vi "20191023_KEK_HEX5_events.vi"() -> ()   [LabVIEW 2017]
uses:
  <vilib>/DAQmx/create/channels.llb/DAQmx Create Channel (AI-Voltage-Basic).vi
  <vilib>/DAQmx/create/channels.llb/DAQmx Create Channel (AO-Voltage-Basic).vi
  <vilib>/DAQmx/miscellaneous.llb/DAQmx Fill In Error Info.vi
  Lake Shore Cryotronics 218.lvlib
panel:
  in  "idx in":i32[](array[numeric])=[0, 1]
  out "Cycle #":i32=68
  out "current time":timestamp=timestamp(3644898422.6679497 s since 1904-01-01)
  in  "stop":bool
  in  "Tab Control":T1(tab)=enum."LSI CHs"
  out "ref LSI-D":refnum<file>
  in  "DAQ IN: P_4HeIN":tag="Dev1/ai16"
  in  "max_P4HeIN":dbl=5.0
  in  "min_P4HeIN":dbl
  in  "DAQ IN: BARA":tag="Dev1/ai7"
  in  "VISA LSI218 DOWN":refnum<visa-resource-name>="GPIB0::11::INSTR"
  in  "DAQ OUT ON?":bool
  out "ref DAQ":refnum<file>
  in  "max_OUT":dbl=5.0
  in  "min_OUT":dbl
  in  "max_FM3":dbl=5.0
  in  "min_FM3":dbl
  in  "max_FM4":dbl=5.0
  in  "min_FM4":dbl
  in  "max_dP3":dbl=5.0
  in  "min_dP3":dbl
  in  "max_dP4":dbl=5.0
  in  "min_dP4":dbl
  in  "max_LM":dbl=0.15
  in  "min_LM":dbl
  in  "max_P":dbl=5.0
  in  "min_P":dbl
  in  "DAQ IN: FM (3He)":tag="Dev1/ai6"
  in  "DAQ IN: FM (4He)":tag="Dev1/ai5"
  in  "DAQ IN: ƒ¢P (3He)":tag="Dev1/ai4"
  in  "DAQ IN: He-level":tag="Dev1/ai2"
  in  "DAQ IN: ƒ¢P (4He)":tag="Dev1/ai3"
  in  "DAQ IN: P (4He coil out)":tag="Dev1/ai1"
  in  "CSV filename suffix":string="TEST_"
  in  "base path":path=path "C:/Users/TUCAN_rcnp/Desktop/Labview/KEK_20191023_HEX5/TEST"
  out "ref LSI-U":refnum<file>
  in  "VISA LSI218 UP":refnum<visa-resource-name>="GPIB0::3::INSTR"
  in  "DAQ OUT":tag="Dev1/ao0"
  in  "sample #":i32=5
  out "error out \n(LSIU)":errorcluster
  out "error out\n(file creation)":errorcluster
  out "error out\n(DAQ config)":errorcluster
  out "error out\n(DAQ OUT)":errorcluster
  out "error out \n(DAQ IN)":errorcluster
  out "error out \n(record LSIU)":errorcluster
  out "error out \n(record DAQ)":errorcluster
  out "error out DAQ close":errorcluster
  out "error out \n(LSID)":errorcluster
  in  "max_BARA":dbl=5.0
  in  "min_BARA":dbl
  in  "min_P3HeOUT":dbl
  in  "max_P3HeOUT":dbl=5.0
  in  "DAQ IN: P_3HeOUT":tag="Dev1/ai17"
  out "error out \n(record LSID)":errorcluster
  out "errors plot cosmetic 1":errorcluster[](array[cluster])
  out "error plot content":errorcluster
  out "error plot cosmetic 2":errorcluster
  in  "LSI-D CH":string[](array[string])=["D1", "D2", "D3", "D4", "D5", "D6", "D7", "D8"]
  in  "NI DAQ AIN labels":string[](array[string])=["P_4KRES_COILIN", "LM", "DP_3He", "DP_4He", "FM_4He", "FM_3He", "P_4KRES_BARA", "P_4He_IN", "P_3He_OUT"]
  in  "LSI-U CH labels":string[](array[string])=["4K_res", "HEX_liq_IN", "HEX_liq_OUT", "1K_pot", "HEX_gas_IN", "HEX_gas_OUT", "JT_IN", "JT_OUT"]
  in  "LSI-D CH labels":string[](array[string])=["D1", "D2", "D3", "DISABLED", "D5", "D6", "D7", "D8"]
  in  "LSI-U CH":string[](array[string])=["U1", "U2", "U3", "U4", "U5", "U6", "U7", "U8"]
  in  "DAQ CH":string[](array[string])=["Q1", "Q2", "Q3", "Q4", "Q5", "Q6", "Q7", "Q8", "Q9"]
  out "D idx":i32[](array[numeric])=[0, 1]
  out "LSI-U CH indic,":string[](array[string])=["U1", "U2", "U3", "U4", "U5", "U6", "U7", "U8"]
  out "LSI-U out":dbl[](array[numeric])=[305.92, 296.12, 291.08, 301.5, 302.08, 302.37, 301.36, 300.38]
  in  "GraphU1 SEL":i32[](array[numeric])=[0, 1]
  out "LSI-D out":dbl[](array[numeric])=[305.92, 296.12, 291.08, 301.5, 302.08, 302.37, 301.36, 300.38]
  out "LSI-D CH indic.":string[](array[string])=["U1", "U2", "U3", "U4", "U5", "U6", "U7", "U8"]
  in  "GraphU2 SEL":i32[](array[numeric])=[2, 3, 4]
  in  "GraphU3 SEL":i32[](array[numeric])=[5, 6, 6]
  in  "GraphD1 SEL":i32[](array[numeric])=[0, 1]
  in  "GraphD2 SEL":i32[](array[numeric])=[2, 3, 4]
  in  "GraphD3 SEL":i32[](array[numeric])=[5, 6, 6]
  out "LSI-D Grpah 1":cluster{dbl[], dbl[]}[](graph)=[{[3644898082.6645026, 3644898087.663789, 3644898092.6640744, 3644898097.66436, 3644898102.6646466, 3644898107.663933, 3644898112.6642184, 3644898117.664504, 3644898122.66379, 3644898127.664076, 3644898132.6643624, 3644898137.665648, 3644898142.6649346, 3644898147.66522, 3644898152.6655064, 3644898157.664792, 3644898162.665078, 3644898167.665364, 3644898172.6656504, 3644898177.664936, 3644898182.665222, 3644898187.665508, 3644898192.6647944, 3644898197.66508, 3644898202.6663666, 3644898207.666652, 3644898212.6659384, 3644898217.666224, 3644898222.6665106, 3644898227.665796, 3644898232.6660824, 3644898237.667368, 3644898242.6676545, 3644898247.66694, 3644898252.6672263, 3644898257.667512, 3644898262.6667986, 3644898267.667084, 3644898272.6673694, 3644898277.667656, 3644898282.6669426, 3644898287.667228, 3644898292.6675134, 3644898297.6678, 3644898302.6680865, 3644898307.668372, 3644898312.668658, 3644898317.667944, 3644898322.6682296, 3644898327.668516, 3644898332.6678014, 3644898337.668088, 3644898342.6683736, 3644898347.66866, 3644898352.6679454, 3644898357.668232, 3644898362.6685176, 3644898367.667804, 3644898372.6680894, 3644898377.668376, 3644898382.6686616, 3644898387.667948, 3644898392.6682334, 3644898397.66852, 3644898402.6678057, 3644898407.6680913, 3644898412.6683774, 3644898417.668664, 3644898422.6679497], [305.66, 305.96, 305.22, 305.33, 305.78, 305.05, 305.43, 306.1, 305.47, 305.83, 305.61, 305.97, 305.69, 305.75, 305.82, 305.82, 305.69, 305.52, 305.52, 306.2, 306.15, 305.92, 305.78, 305.61, 305.73, 305.41, 305.57, 306.24, 306.43, 305.83, 305.97, 306.01, 306.34, 305.78, 305.78, 306.48, 306.2, 306.2, 305.47, 305.96, 305.57, 305.97, 305.83, 305.83, 306.06, 305.92, 305.66, 305.82, 305.64, 305.57, 305.78, 305.73, 306.17, 305.83, 305.9, 306.15, 305.43, 305.87, 306.24, 306.04, 305.82, 306.06, 305.52, 305.75, 306.04, 306.06, 305.48, 305.75, 305.92]}, {[3644898082.6645026, 3644898087.663789, 3644898092.6640744, 3644898097.66436, 3644898102.6646466, 3644898107.663933, 3644898112.6642184, 3644898117.664504, 3644898122.66379, 3644898127.664076, 3644898132.6643624, 3644898137.665648, 3644898142.6649346, 3644898147.66522, 3644898152.6655064, 3644898157.664792, 3644898162.665078, 3644898167.665364, 3644898172.6656504, 3644898177.664936, 3644898182.665222, 3644898187.665508, 3644898192.6647944, 3644898197.66508, 3644898202.6663666, 3644898207.666652, 3644898212.6659384, 3644898217.666224, 3644898222.6665106, 3644898227.665796, 3644898232.6660824, 3644898237.667368, 3644898242.6676545, 3644898247.66694, 3644898252.6672263, 3644898257.667512, 3644898262.6667986, 3644898267.667084, 3644898272.6673694, 3644898277.667656, 3644898282.6669426, 3644898287.667228, 3644898292.6675134, 3644898297.6678, 3644898302.6680865, 3644898307.668372, 3644898312.668658, 3644898317.667944, 3644898322.6682296, 3644898327.668516, 3644898332.6678014, 3644898337.668088, 3644898342.6683736, 3644898347.66866, 3644898352.6679454, 3644898357.668232, 3644898362.6685176, 3644898367.667804, 3644898372.6680894, 3644898377.668376, 3644898382.6686616, 3644898387.667948, 3644898392.6682334, 3644898397.66852, 3644898402.6678057, 3644898407.6680913, 3644898412.6683774, 3644898417.668664, 3644898422.6679497], [296.0, 296.1, 295.89, 295.78, 295.94, 295.91, 295.97, 296.12, 296.01, 296.1, 296.01, 296.2, 296.14, 296.06, 296.16, 296.08, 295.89, 295.97, 296.06, 296.03, 296.09, 295.99, 295.89, 295.85, 295.93, 295.74, 295.91, 296.21, 296.04, 296.14, 296.12, 295.91, 296.2, 295.91, 295.87, 296.09, 296.19, 295.91, 296.03, 296.12, 295.94, 296.03, 295.97, 296.01, 296.08, 295.89, 295.91, 295.97, 296.03, 295.81, 295.91, 296.1, 296.15, 296.05, 296.15, 296.24, 295.82, 295.81, 296.14, 296.24, 295.97, 296.06, 295.74, 295.95, 296.08, 295.94, 295.91, 295.91, 296.12]}, {[3644898082.6645026, 3644898087.663789, 3644898092.6640744, 3644898097.66436, 3644898102.6646466, 3644898107.663933, 3644898112.6642184, 3644898117.664504, 3644898122.66379, 3644898127.664076, 3644898132.6643624, 3644898137.665648, 3644898142.6649346, 3644898147.66522, 3644898152.6655064, 3644898157.664792, 3644898162.665078, 3644898167.665364, 3644898172.6656504, 3644898177.664936, 3644898182.665222, 3644898187.665508, 3644898192.6647944, 3644898197.66508, 3644898202.6663666, 3644898207.666652, 3644898212.6659384, 3644898217.666224, 3644898222.6665106, 3644898227.665796, 3644898232.6660824, 3644898237.667368, 3644898242.6676545, 3644898247.66694, 3644898252.6672263, 3644898257.667512, 3644898262.6667986, 3644898267.667084, 3644898272.6673694, 3644898277.667656, 3644898282.6669426, 3644898287.667228, 3644898292.6675134, 3644898297.6678, 3644898302.6680865, 3644898307.668372, 3644898312.668658, 3644898317.667944, 3644898322.6682296, 3644898327.668516, 3644898332.6678014, 3644898337.668088, 3644898342.6683736, 3644898347.66866, 3644898352.6679454, 3644898357.668232, 3644898362.6685176, 3644898367.667804, 3644898372.6680894, 3644898377.668376, 3644898382.6686616, 3644898387.667948, 3644898392.6682334, 3644898397.66852, 3644898402.6678057, 3644898407.6680913, 3644898412.6683774, 3644898417.668664, 3644898422.6679497], [290.48, 291.09, 290.9, 291.1, 290.9, 290.9, 291.04, 291.04, 290.99, 290.93, 290.9, 291.31, 290.97, 291.13, 291.04, 291.12, 290.93, 290.69, 291.06, 291.27, 291.06, 291.04, 290.96, 291.09, 290.86, 290.95, 291.01, 291.18, 291.25, 291.18, 290.95, 291.08, 291.12, 290.97, 290.93, 291.09, 291.27, 291.02, 290.93, 291.08, 291.22, 291.12, 290.92, 290.69, 291.02, 291.02, 290.9, 290.86, 291.08, 290.88, 290.77, 291.01, 291.05, 291.1, 291.14, 290.99, 291.06, 290.9, 291.05, 291.31, 291.05, 291.06, 290.95, 290.99, 290.99, 290.9, 290.9, 290.96, 291.08]}]
  out "LSI-U Grpah 1":cluster{dbl[], dbl[]}[](graph)=[{[3644898082.6645026, 3644898087.663789, 3644898092.6640744, 3644898097.66436, 3644898102.6646466, 3644898107.663933, 3644898112.6642184, 3644898117.664504, 3644898122.66379, 3644898127.664076, 3644898132.6643624, 3644898137.665648, 3644898142.6649346, 3644898147.66522, 3644898152.6655064, 3644898157.664792, 3644898162.665078, 3644898167.665364, 3644898172.6656504, 3644898177.664936, 3644898182.665222, 3644898187.665508, 3644898192.6647944, 3644898197.66508, 3644898202.6663666, 3644898207.666652, 3644898212.6659384, 3644898217.666224, 3644898222.6665106, 3644898227.665796, 3644898232.6660824, 3644898237.667368, 3644898242.6676545, 3644898247.66694, 3644898252.6672263, 3644898257.667512, 3644898262.6667986, 3644898267.667084, 3644898272.6673694, 3644898277.667656, 3644898282.6669426, 3644898287.667228, 3644898292.6675134, 3644898297.6678, 3644898302.6680865, 3644898307.668372, 3644898312.668658, 3644898317.667944, 3644898322.6682296, 3644898327.668516, 3644898332.6678014, 3644898337.668088, 3644898342.6683736, 3644898347.66866, 3644898352.6679454, 3644898357.668232, 3644898362.6685176, 3644898367.667804, 3644898372.6680894, 3644898377.668376, 3644898382.6686616, 3644898387.667948, 3644898392.6682334, 3644898397.66852, 3644898402.6678057, 3644898407.6680913, 3644898412.6683774, 3644898417.668664, 3644898422.6679497], [305.66, 305.96, 305.22, 305.33, 305.78, 305.05, 305.43, 306.1, 305.47, 305.83, 305.61, 305.97, 305.69, 305.75, 305.82, 305.82, 305.69, 305.52, 305.52, 306.2, 306.15, 305.92, 305.78, 305.61, 305.73, 305.41, 305.57, 306.24, 306.43, 305.83, 305.97, 306.01, 306.34, 305.78, 305.78, 306.48, 306.2, 306.2, 305.47, 305.96, 305.57, 305.97, 305.83, 305.83, 306.06, 305.92, 305.66, 305.82, 305.64, 305.57, 305.78, 305.73, 306.17, 305.83, 305.9, 306.15, 305.43, 305.87, 306.24, 306.04, 305.82, 306.06, 305.52, 305.75, 306.04, 306.06, 305.48, 305.75, 305.92]}, {[3644898082.6645026, 3644898087.663789, 3644898092.6640744, 3644898097.66436, 3644898102.6646466, 3644898107.663933, 3644898112.6642184, 3644898117.664504, 3644898122.66379, 3644898127.664076, 3644898132.6643624, 3644898137.665648, 3644898142.6649346, 3644898147.66522, 3644898152.6655064, 3644898157.664792, 3644898162.665078, 3644898167.665364, 3644898172.6656504, 3644898177.664936, 3644898182.665222, 3644898187.665508, 3644898192.6647944, 3644898197.66508, 3644898202.6663666, 3644898207.666652, 3644898212.6659384, 3644898217.666224, 3644898222.6665106, 3644898227.665796, 3644898232.6660824, 3644898237.667368, 3644898242.6676545, 3644898247.66694, 3644898252.6672263, 3644898257.667512, 3644898262.6667986, 3644898267.667084, 3644898272.6673694, 3644898277.667656, 3644898282.6669426, 3644898287.667228, 3644898292.6675134, 3644898297.6678, 3644898302.6680865, 3644898307.668372, 3644898312.668658, 3644898317.667944, 3644898322.6682296, 3644898327.668516, 3644898332.6678014, 3644898337.668088, 3644898342.6683736, 3644898347.66866, 3644898352.6679454, 3644898357.668232, 3644898362.6685176, 3644898367.667804, 3644898372.6680894, 3644898377.668376, 3644898382.6686616, 3644898387.667948, 3644898392.6682334, 3644898397.66852, 3644898402.6678057, 3644898407.6680913, 3644898412.6683774, 3644898417.668664, 3644898422.6679497], [296.0, 296.1, 295.89, 295.78, 295.94, 295.91, 295.97, 296.12, 296.01, 296.1, 296.01, 296.2, 296.14, 296.06, 296.16, 296.08, 295.89, 295.97, 296.06, 296.03, 296.09, 295.99, 295.89, 295.85, 295.93, 295.74, 295.91, 296.21, 296.04, 296.14, 296.12, 295.91, 296.2, 295.91, 295.87, 296.09, 296.19, 295.91, 296.03, 296.12, 295.94, 296.03, 295.97, 296.01, 296.08, 295.89, 295.91, 295.97, 296.03, 295.81, 295.91, 296.1, 296.15, 296.05, 296.15, 296.24, 295.82, 295.81, 296.14, 296.24, 295.97, 296.06, 295.74, 295.95, 296.08, 295.94, 295.91, 295.91, 296.12]}, {[3644898082.6645026, 3644898087.663789, 3644898092.6640744, 3644898097.66436, 3644898102.6646466, 3644898107.663933, 3644898112.6642184, 3644898117.664504, 3644898122.66379, 3644898127.664076, 3644898132.6643624, 3644898137.665648, 3644898142.6649346, 3644898147.66522, 3644898152.6655064, 3644898157.664792, 3644898162.665078, 3644898167.665364, 3644898172.6656504, 3644898177.664936, 3644898182.665222, 3644898187.665508, 3644898192.6647944, 3644898197.66508, 3644898202.6663666, 3644898207.666652, 3644898212.6659384, 3644898217.666224, 3644898222.6665106, 3644898227.665796, 3644898232.6660824, 3644898237.667368, 3644898242.6676545, 3644898247.66694, 3644898252.6672263, 3644898257.667512, 3644898262.6667986, 3644898267.667084, 3644898272.6673694, 3644898277.667656, 3644898282.6669426, 3644898287.667228, 3644898292.6675134, 3644898297.6678, 3644898302.6680865, 3644898307.668372, 3644898312.668658, 3644898317.667944, 3644898322.6682296, 3644898327.668516, 3644898332.6678014, 3644898337.668088, 3644898342.6683736, 3644898347.66866, 3644898352.6679454, 3644898357.668232, 3644898362.6685176, 3644898367.667804, 3644898372.6680894, 3644898377.668376, 3644898382.6686616, 3644898387.667948, 3644898392.6682334, 3644898397.66852, 3644898402.6678057, 3644898407.6680913, 3644898412.6683774, 3644898417.668664, 3644898422.6679497], [290.48, 291.09, 290.9, 291.1, 290.9, 290.9, 291.04, 291.04, 290.99, 290.93, 290.9, 291.31, 290.97, 291.13, 291.04, 291.12, 290.93, 290.69, 291.06, 291.27, 291.06, 291.04, 290.96, 291.09, 290.86, 290.95, 291.01, 291.18, 291.25, 291.18, 290.95, 291.08, 291.12, 290.97, 290.93, 291.09, 291.27, 291.02, 290.93, 291.08, 291.22, 291.12, 290.92, 290.69, 291.02, 291.02, 290.9, 290.86, 291.08, 290.88, 290.77, 291.01, 291.05, 291.1, 291.14, 290.99, 291.06, 290.9, 291.05, 291.31, 291.05, 291.06, 290.95, 290.99, 290.99, 290.9, 290.9, 290.96, 291.08]}]
  out "LSI-D Grpah 2":cluster{dbl[], dbl[]}[](graph)=[{[3644898082.6645026, 3644898087.663789, 3644898092.6640744, 3644898097.66436, 3644898102.6646466, 3644898107.663933, 3644898112.6642184, 3644898117.664504, 3644898122.66379, 3644898127.664076, 3644898132.6643624, 3644898137.665648, 3644898142.6649346, 3644898147.66522, 3644898152.6655064, 3644898157.664792, 3644898162.665078, 3644898167.665364, 3644898172.6656504, 3644898177.664936, 3644898182.665222, 3644898187.665508, 3644898192.6647944, 3644898197.66508, 3644898202.6663666, 3644898207.666652, 3644898212.6659384, 3644898217.666224, 3644898222.6665106, 3644898227.665796, 3644898232.6660824, 3644898237.667368, 3644898242.6676545, 3644898247.66694, 3644898252.6672263, 3644898257.667512, 3644898262.6667986, 3644898267.667084, 3644898272.6673694, 3644898277.667656, 3644898282.6669426, 3644898287.667228, 3644898292.6675134, 3644898297.6678, 3644898302.6680865, 3644898307.668372, 3644898312.668658, 3644898317.667944, 3644898322.6682296, 3644898327.668516, 3644898332.6678014, 3644898337.668088, 3644898342.6683736, 3644898347.66866, 3644898352.6679454, 3644898357.668232, 3644898362.6685176, 3644898367.667804, 3644898372.6680894, 3644898377.668376, 3644898382.6686616, 3644898387.667948, 3644898392.6682334, 3644898397.66852, 3644898402.6678057, 3644898407.6680913, 3644898412.6683774, 3644898417.668664, 3644898422.6679497], [305.66, 305.96, 305.22, 305.33, 305.78, 305.05, 305.43, 306.1, 305.47, 305.83, 305.61, 305.97, 305.69, 305.75, 305.82, 305.82, 305.69, 305.52, 305.52, 306.2, 306.15, 305.92, 305.78, 305.61, 305.73, 305.41, 305.57, 306.24, 306.43, 305.83, 305.97, 306.01, 306.34, 305.78, 305.78, 306.48, 306.2, 306.2, 305.47, 305.96, 305.57, 305.97, 305.83, 305.83, 306.06, 305.92, 305.66, 305.82, 305.64, 305.57, 305.78, 305.73, 306.17, 305.83, 305.9, 306.15, 305.43, 305.87, 306.24, 306.04, 305.82, 306.06, 305.52, 305.75, 306.04, 306.06, 305.48, 305.75, 305.92]}, {[3644898082.6645026, 3644898087.663789, 3644898092.6640744, 3644898097.66436, 3644898102.6646466, 3644898107.663933, 3644898112.6642184, 3644898117.664504, 3644898122.66379, 3644898127.664076, 3644898132.6643624, 3644898137.665648, 3644898142.6649346, 3644898147.66522, 3644898152.6655064, 3644898157.664792, 3644898162.665078, 3644898167.665364, 3644898172.6656504, 3644898177.664936, 3644898182.665222, 3644898187.665508, 3644898192.6647944, 3644898197.66508, 3644898202.6663666, 3644898207.666652, 3644898212.6659384, 3644898217.666224, 3644898222.6665106, 3644898227.665796, 3644898232.6660824, 3644898237.667368, 3644898242.6676545, 3644898247.66694, 3644898252.6672263, 3644898257.667512, 3644898262.6667986, 3644898267.667084, 3644898272.6673694, 3644898277.667656, 3644898282.6669426, 3644898287.667228, 3644898292.6675134, 3644898297.6678, 3644898302.6680865, 3644898307.668372, 3644898312.668658, 3644898317.667944, 3644898322.6682296, 3644898327.668516, 3644898332.6678014, 3644898337.668088, 3644898342.6683736, 3644898347.66866, 3644898352.6679454, 3644898357.668232, 3644898362.6685176, 3644898367.667804, 3644898372.6680894, 3644898377.668376, 3644898382.6686616, 3644898387.667948, 3644898392.6682334, 3644898397.66852, 3644898402.6678057, 3644898407.6680913, 3644898412.6683774, 3644898417.668664, 3644898422.6679497], [296.0, 296.1, 295.89, 295.78, 295.94, 295.91, 295.97, 296.12, 296.01, 296.1, 296.01, 296.2, 296.14, 296.06, 296.16, 296.08, 295.89, 295.97, 296.06, 296.03, 296.09, 295.99, 295.89, 295.85, 295.93, 295.74, 295.91, 296.21, 296.04, 296.14, 296.12, 295.91, 296.2, 295.91, 295.87, 296.09, 296.19, 295.91, 296.03, 296.12, 295.94, 296.03, 295.97, 296.01, 296.08, 295.89, 295.91, 295.97, 296.03, 295.81, 295.91, 296.1, 296.15, 296.05, 296.15, 296.24, 295.82, 295.81, 296.14, 296.24, 295.97, 296.06, 295.74, 295.95, 296.08, 295.94, 295.91, 295.91, 296.12]}, {[3644898082.6645026, 3644898087.663789, 3644898092.6640744, 3644898097.66436, 3644898102.6646466, 3644898107.663933, 3644898112.6642184, 3644898117.664504, 3644898122.66379, 3644898127.664076, 3644898132.6643624, 3644898137.665648, 3644898142.6649346, 3644898147.66522, 3644898152.6655064, 3644898157.664792, 3644898162.665078, 3644898167.665364, 3644898172.6656504, 3644898177.664936, 3644898182.665222, 3644898187.665508, 3644898192.6647944, 3644898197.66508, 3644898202.6663666, 3644898207.666652, 3644898212.6659384, 3644898217.666224, 3644898222.6665106, 3644898227.665796, 3644898232.6660824, 3644898237.667368, 3644898242.6676545, 3644898247.66694, 3644898252.6672263, 3644898257.667512, 3644898262.6667986, 3644898267.667084, 3644898272.6673694, 3644898277.667656, 3644898282.6669426, 3644898287.667228, 3644898292.6675134, 3644898297.6678, 3644898302.6680865, 3644898307.668372, 3644898312.668658, 3644898317.667944, 3644898322.6682296, 3644898327.668516, 3644898332.6678014, 3644898337.668088, 3644898342.6683736, 3644898347.66866, 3644898352.6679454, 3644898357.668232, 3644898362.6685176, 3644898367.667804, 3644898372.6680894, 3644898377.668376, 3644898382.6686616, 3644898387.667948, 3644898392.6682334, 3644898397.66852, 3644898402.6678057, 3644898407.6680913, 3644898412.6683774, 3644898417.668664, 3644898422.6679497], [290.48, 291.09, 290.9, 291.1, 290.9, 290.9, 291.04, 291.04, 290.99, 290.93, 290.9, 291.31, 290.97, 291.13, 291.04, 291.12, 290.93, 290.69, 291.06, 291.27, 291.06, 291.04, 290.96, 291.09, 290.86, 290.95, 291.01, 291.18, 291.25, 291.18, 290.95, 291.08, 291.12, 290.97, 290.93, 291.09, 291.27, 291.02, 290.93, 291.08, 291.22, 291.12, 290.92, 290.69, 291.02, 291.02, 290.9, 290.86, 291.08, 290.88, 290.77, 291.01, 291.05, 291.1, 291.14, 290.99, 291.06, 290.9, 291.05, 291.31, 291.05, 291.06, 290.95, 290.99, 290.99, 290.9, 290.9, 290.96, 291.08]}]
  out "LSI-U Grpah 3":cluster{dbl[], dbl[]}[](graph)=[{[3644898082.6645026, 3644898087.663789, 3644898092.6640744, 3644898097.66436, 3644898102.6646466, 3644898107.663933, 3644898112.6642184, 3644898117.664504, 3644898122.66379, 3644898127.664076, 3644898132.6643624, 3644898137.665648, 3644898142.6649346, 3644898147.66522, 3644898152.6655064, 3644898157.664792, 3644898162.665078, 3644898167.665364, 3644898172.6656504, 3644898177.664936, 3644898182.665222, 3644898187.665508, 3644898192.6647944, 3644898197.66508, 3644898202.6663666, 3644898207.666652, 3644898212.6659384, 3644898217.666224, 3644898222.6665106, 3644898227.665796, 3644898232.6660824, 3644898237.667368, 3644898242.6676545, 3644898247.66694, 3644898252.6672263, 3644898257.667512, 3644898262.6667986, 3644898267.667084, 3644898272.6673694, 3644898277.667656, 3644898282.6669426, 3644898287.667228, 3644898292.6675134, 3644898297.6678, 3644898302.6680865, 3644898307.668372, 3644898312.668658, 3644898317.667944, 3644898322.6682296, 3644898327.668516, 3644898332.6678014, 3644898337.668088, 3644898342.6683736, 3644898347.66866, 3644898352.6679454, 3644898357.668232, 3644898362.6685176, 3644898367.667804, 3644898372.6680894, 3644898377.668376, 3644898382.6686616, 3644898387.667948, 3644898392.6682334, 3644898397.66852, 3644898402.6678057, 3644898407.6680913, 3644898412.6683774, 3644898417.668664, 3644898422.6679497], [305.66, 305.96, 305.22, 305.33, 305.78, 305.05, 305.43, 306.1, 305.47, 305.83, 305.61, 305.97, 305.69, 305.75, 305.82, 305.82, 305.69, 305.52, 305.52, 306.2, 306.15, 305.92, 305.78, 305.61, 305.73, 305.41, 305.57, 306.24, 306.43, 305.83, 305.97, 306.01, 306.34, 305.78, 305.78, 306.48, 306.2, 306.2, 305.47, 305.96, 305.57, 305.97, 305.83, 305.83, 306.06, 305.92, 305.66, 305.82, 305.64, 305.57, 305.78, 305.73, 306.17, 305.83, 305.9, 306.15, 305.43, 305.87, 306.24, 306.04, 305.82, 306.06, 305.52, 305.75, 306.04, 306.06, 305.48, 305.75, 305.92]}, {[3644898082.6645026, 3644898087.663789, 3644898092.6640744, 3644898097.66436, 3644898102.6646466, 3644898107.663933, 3644898112.6642184, 3644898117.664504, 3644898122.66379, 3644898127.664076, 3644898132.6643624, 3644898137.665648, 3644898142.6649346, 3644898147.66522, 3644898152.6655064, 3644898157.664792, 3644898162.665078, 3644898167.665364, 3644898172.6656504, 3644898177.664936, 3644898182.665222, 3644898187.665508, 3644898192.6647944, 3644898197.66508, 3644898202.6663666, 3644898207.666652, 3644898212.6659384, 3644898217.666224, 3644898222.6665106, 3644898227.665796, 3644898232.6660824, 3644898237.667368, 3644898242.6676545, 3644898247.66694, 3644898252.6672263, 3644898257.667512, 3644898262.6667986, 3644898267.667084, 3644898272.6673694, 3644898277.667656, 3644898282.6669426, 3644898287.667228, 3644898292.6675134, 3644898297.6678, 3644898302.6680865, 3644898307.668372, 3644898312.668658, 3644898317.667944, 3644898322.6682296, 3644898327.668516, 3644898332.6678014, 3644898337.668088, 3644898342.6683736, 3644898347.66866, 3644898352.6679454, 3644898357.668232, 3644898362.6685176, 3644898367.667804, 3644898372.6680894, 3644898377.668376, 3644898382.6686616, 3644898387.667948, 3644898392.6682334, 3644898397.66852, 3644898402.6678057, 3644898407.6680913, 3644898412.6683774, 3644898417.668664, 3644898422.6679497], [296.0, 296.1, 295.89, 295.78, 295.94, 295.91, 295.97, 296.12, 296.01, 296.1, 296.01, 296.2, 296.14, 296.06, 296.16, 296.08, 295.89, 295.97, 296.06, 296.03, 296.09, 295.99, 295.89, 295.85, 295.93, 295.74, 295.91, 296.21, 296.04, 296.14, 296.12, 295.91, 296.2, 295.91, 295.87, 296.09, 296.19, 295.91, 296.03, 296.12, 295.94, 296.03, 295.97, 296.01, 296.08, 295.89, 295.91, 295.97, 296.03, 295.81, 295.91, 296.1, 296.15, 296.05, 296.15, 296.24, 295.82, 295.81, 296.14, 296.24, 295.97, 296.06, 295.74, 295.95, 296.08, 295.94, 295.91, 295.91, 296.12]}, {[3644898082.6645026, 3644898087.663789, 3644898092.6640744, 3644898097.66436, 3644898102.6646466, 3644898107.663933, 3644898112.6642184, 3644898117.664504, 3644898122.66379, 3644898127.664076, 3644898132.6643624, 3644898137.665648, 3644898142.6649346, 3644898147.66522, 3644898152.6655064, 3644898157.664792, 3644898162.665078, 3644898167.665364, 3644898172.6656504, 3644898177.664936, 3644898182.665222, 3644898187.665508, 3644898192.6647944, 3644898197.66508, 3644898202.6663666, 3644898207.666652, 3644898212.6659384, 3644898217.666224, 3644898222.6665106, 3644898227.665796, 3644898232.6660824, 3644898237.667368, 3644898242.6676545, 3644898247.66694, 3644898252.6672263, 3644898257.667512, 3644898262.6667986, 3644898267.667084, 3644898272.6673694, 3644898277.667656, 3644898282.6669426, 3644898287.667228, 3644898292.6675134, 3644898297.6678, 3644898302.6680865, 3644898307.668372, 3644898312.668658, 3644898317.667944, 3644898322.6682296, 3644898327.668516, 3644898332.6678014, 3644898337.668088, 3644898342.6683736, 3644898347.66866, 3644898352.6679454, 3644898357.668232, 3644898362.6685176, 3644898367.667804, 3644898372.6680894, 3644898377.668376, 3644898382.6686616, 3644898387.667948, 3644898392.6682334, 3644898397.66852, 3644898402.6678057, 3644898407.6680913, 3644898412.6683774, 3644898417.668664, 3644898422.6679497], [290.48, 291.09, 290.9, 291.1, 290.9, 290.9, 291.04, 291.04, 290.99, 290.93, 290.9, 291.31, 290.97, 291.13, 291.04, 291.12, 290.93, 290.69, 291.06, 291.27, 291.06, 291.04, 290.96, 291.09, 290.86, 290.95, 291.01, 291.18, 291.25, 291.18, 290.95, 291.08, 291.12, 290.97, 290.93, 291.09, 291.27, 291.02, 290.93, 291.08, 291.22, 291.12, 290.92, 290.69, 291.02, 291.02, 290.9, 290.86, 291.08, 290.88, 290.77, 291.01, 291.05, 291.1, 291.14, 290.99, 291.06, 290.9, 291.05, 291.31, 291.05, 291.06, 290.95, 290.99, 290.99, 290.9, 290.9, 290.96, 291.08]}]
  out "LSI-U Grpah 2":cluster{dbl[], dbl[]}[](graph)=[{[3644898082.6645026, 3644898087.663789, 3644898092.6640744, 3644898097.66436, 3644898102.6646466, 3644898107.663933, 3644898112.6642184, 3644898117.664504, 3644898122.66379, 3644898127.664076, 3644898132.6643624, 3644898137.665648, 3644898142.6649346, 3644898147.66522, 3644898152.6655064, 3644898157.664792, 3644898162.665078, 3644898167.665364, 3644898172.6656504, 3644898177.664936, 3644898182.665222, 3644898187.665508, 3644898192.6647944, 3644898197.66508, 3644898202.6663666, 3644898207.666652, 3644898212.6659384, 3644898217.666224, 3644898222.6665106, 3644898227.665796, 3644898232.6660824, 3644898237.667368, 3644898242.6676545, 3644898247.66694, 3644898252.6672263, 3644898257.667512, 3644898262.6667986, 3644898267.667084, 3644898272.6673694, 3644898277.667656, 3644898282.6669426, 3644898287.667228, 3644898292.6675134, 3644898297.6678, 3644898302.6680865, 3644898307.668372, 3644898312.668658, 3644898317.667944, 3644898322.6682296, 3644898327.668516, 3644898332.6678014, 3644898337.668088, 3644898342.6683736, 3644898347.66866, 3644898352.6679454, 3644898357.668232, 3644898362.6685176, 3644898367.667804, 3644898372.6680894, 3644898377.668376, 3644898382.6686616, 3644898387.667948, 3644898392.6682334, 3644898397.66852, 3644898402.6678057, 3644898407.6680913, 3644898412.6683774, 3644898417.668664, 3644898422.6679497], [305.66, 305.96, 305.22, 305.33, 305.78, 305.05, 305.43, 306.1, 305.47, 305.83, 305.61, 305.97, 305.69, 305.75, 305.82, 305.82, 305.69, 305.52, 305.52, 306.2, 306.15, 305.92, 305.78, 305.61, 305.73, 305.41, 305.57, 306.24, 306.43, 305.83, 305.97, 306.01, 306.34, 305.78, 305.78, 306.48, 306.2, 306.2, 305.47, 305.96, 305.57, 305.97, 305.83, 305.83, 306.06, 305.92, 305.66, 305.82, 305.64, 305.57, 305.78, 305.73, 306.17, 305.83, 305.9, 306.15, 305.43, 305.87, 306.24, 306.04, 305.82, 306.06, 305.52, 305.75, 306.04, 306.06, 305.48, 305.75, 305.92]}, {[3644898082.6645026, 3644898087.663789, 3644898092.6640744, 3644898097.66436, 3644898102.6646466, 3644898107.663933, 3644898112.6642184, 3644898117.664504, 3644898122.66379, 3644898127.664076, 3644898132.6643624, 3644898137.665648, 3644898142.6649346, 3644898147.66522, 3644898152.6655064, 3644898157.664792, 3644898162.665078, 3644898167.665364, 3644898172.6656504, 3644898177.664936, 3644898182.665222, 3644898187.665508, 3644898192.6647944, 3644898197.66508, 3644898202.6663666, 3644898207.666652, 3644898212.6659384, 3644898217.666224, 3644898222.6665106, 3644898227.665796, 3644898232.6660824, 3644898237.667368, 3644898242.6676545, 3644898247.66694, 3644898252.6672263, 3644898257.667512, 3644898262.6667986, 3644898267.667084, 3644898272.6673694, 3644898277.667656, 3644898282.6669426, 3644898287.667228, 3644898292.6675134, 3644898297.6678, 3644898302.6680865, 3644898307.668372, 3644898312.668658, 3644898317.667944, 3644898322.6682296, 3644898327.668516, 3644898332.6678014, 3644898337.668088, 3644898342.6683736, 3644898347.66866, 3644898352.6679454, 3644898357.668232, 3644898362.6685176, 3644898367.667804, 3644898372.6680894, 3644898377.668376, 3644898382.6686616, 3644898387.667948, 3644898392.6682334, 3644898397.66852, 3644898402.6678057, 3644898407.6680913, 3644898412.6683774, 3644898417.668664, 3644898422.6679497], [296.0, 296.1, 295.89, 295.78, 295.94, 295.91, 295.97, 296.12, 296.01, 296.1, 296.01, 296.2, 296.14, 296.06, 296.16, 296.08, 295.89, 295.97, 296.06, 296.03, 296.09, 295.99, 295.89, 295.85, 295.93, 295.74, 295.91, 296.21, 296.04, 296.14, 296.12, 295.91, 296.2, 295.91, 295.87, 296.09, 296.19, 295.91, 296.03, 296.12, 295.94, 296.03, 295.97, 296.01, 296.08, 295.89, 295.91, 295.97, 296.03, 295.81, 295.91, 296.1, 296.15, 296.05, 296.15, 296.24, 295.82, 295.81, 296.14, 296.24, 295.97, 296.06, 295.74, 295.95, 296.08, 295.94, 295.91, 295.91, 296.12]}, {[3644898082.6645026, 3644898087.663789, 3644898092.6640744, 3644898097.66436, 3644898102.6646466, 3644898107.663933, 3644898112.6642184, 3644898117.664504, 3644898122.66379, 3644898127.664076, 3644898132.6643624, 3644898137.665648, 3644898142.6649346, 3644898147.66522, 3644898152.6655064, 3644898157.664792, 3644898162.665078, 3644898167.665364, 3644898172.6656504, 3644898177.664936, 3644898182.665222, 3644898187.665508, 3644898192.6647944, 3644898197.66508, 3644898202.6663666, 3644898207.666652, 3644898212.6659384, 3644898217.666224, 3644898222.6665106, 3644898227.665796, 3644898232.6660824, 3644898237.667368, 3644898242.6676545, 3644898247.66694, 3644898252.6672263, 3644898257.667512, 3644898262.6667986, 3644898267.667084, 3644898272.6673694, 3644898277.667656, 3644898282.6669426, 3644898287.667228, 3644898292.6675134, 3644898297.6678, 3644898302.6680865, 3644898307.668372, 3644898312.668658, 3644898317.667944, 3644898322.6682296, 3644898327.668516, 3644898332.6678014, 3644898337.668088, 3644898342.6683736, 3644898347.66866, 3644898352.6679454, 3644898357.668232, 3644898362.6685176, 3644898367.667804, 3644898372.6680894, 3644898377.668376, 3644898382.6686616, 3644898387.667948, 3644898392.6682334, 3644898397.66852, 3644898402.6678057, 3644898407.6680913, 3644898412.6683774, 3644898417.668664, 3644898422.6679497], [290.48, 291.09, 290.9, 291.1, 290.9, 290.9, 291.04, 291.04, 290.99, 290.93, 290.9, 291.31, 290.97, 291.13, 291.04, 291.12, 290.93, 290.69, 291.06, 291.27, 291.06, 291.04, 290.96, 291.09, 290.86, 290.95, 291.01, 291.18, 291.25, 291.18, 290.95, 291.08, 291.12, 290.97, 290.93, 291.09, 291.27, 291.02, 290.93, 291.08, 291.22, 291.12, 290.92, 290.69, 291.02, 291.02, 290.9, 290.86, 291.08, 290.88, 290.77, 291.01, 291.05, 291.1, 291.14, 290.99, 291.06, 290.9, 291.05, 291.31, 291.05, 291.06, 290.95, 290.99, 290.99, 290.9, 290.9, 290.96, 291.08]}]
  out "LSI-D Grpah 3":cluster{dbl[], dbl[]}[](graph)=[{[3644898082.6645026, 3644898087.663789, 3644898092.6640744, 3644898097.66436, 3644898102.6646466, 3644898107.663933, 3644898112.6642184, 3644898117.664504, 3644898122.66379, 3644898127.664076, 3644898132.6643624, 3644898137.665648, 3644898142.6649346, 3644898147.66522, 3644898152.6655064, 3644898157.664792, 3644898162.665078, 3644898167.665364, 3644898172.6656504, 3644898177.664936, 3644898182.665222, 3644898187.665508, 3644898192.6647944, 3644898197.66508, 3644898202.6663666, 3644898207.666652, 3644898212.6659384, 3644898217.666224, 3644898222.6665106, 3644898227.665796, 3644898232.6660824, 3644898237.667368, 3644898242.6676545, 3644898247.66694, 3644898252.6672263, 3644898257.667512, 3644898262.6667986, 3644898267.667084, 3644898272.6673694, 3644898277.667656, 3644898282.6669426, 3644898287.667228, 3644898292.6675134, 3644898297.6678, 3644898302.6680865, 3644898307.668372, 3644898312.668658, 3644898317.667944, 3644898322.6682296, 3644898327.668516, 3644898332.6678014, 3644898337.668088, 3644898342.6683736, 3644898347.66866, 3644898352.6679454, 3644898357.668232, 3644898362.6685176, 3644898367.667804, 3644898372.6680894, 3644898377.668376, 3644898382.6686616, 3644898387.667948, 3644898392.6682334, 3644898397.66852, 3644898402.6678057, 3644898407.6680913, 3644898412.6683774, 3644898417.668664, 3644898422.6679497], [305.66, 305.96, 305.22, 305.33, 305.78, 305.05, 305.43, 306.1, 305.47, 305.83, 305.61, 305.97, 305.69, 305.75, 305.82, 305.82, 305.69, 305.52, 305.52, 306.2, 306.15, 305.92, 305.78, 305.61, 305.73, 305.41, 305.57, 306.24, 306.43, 305.83, 305.97, 306.01, 306.34, 305.78, 305.78, 306.48, 306.2, 306.2, 305.47, 305.96, 305.57, 305.97, 305.83, 305.83, 306.06, 305.92, 305.66, 305.82, 305.64, 305.57, 305.78, 305.73, 306.17, 305.83, 305.9, 306.15, 305.43, 305.87, 306.24, 306.04, 305.82, 306.06, 305.52, 305.75, 306.04, 306.06, 305.48, 305.75, 305.92]}, {[3644898082.6645026, 3644898087.663789, 3644898092.6640744, 3644898097.66436, 3644898102.6646466, 3644898107.663933, 3644898112.6642184, 3644898117.664504, 3644898122.66379, 3644898127.664076, 3644898132.6643624, 3644898137.665648, 3644898142.6649346, 3644898147.66522, 3644898152.6655064, 3644898157.664792, 3644898162.665078, 3644898167.665364, 3644898172.6656504, 3644898177.664936, 3644898182.665222, 3644898187.665508, 3644898192.6647944, 3644898197.66508, 3644898202.6663666, 3644898207.666652, 3644898212.6659384, 3644898217.666224, 3644898222.6665106, 3644898227.665796, 3644898232.6660824, 3644898237.667368, 3644898242.6676545, 3644898247.66694, 3644898252.6672263, 3644898257.667512, 3644898262.6667986, 3644898267.667084, 3644898272.6673694, 3644898277.667656, 3644898282.6669426, 3644898287.667228, 3644898292.6675134, 3644898297.6678, 3644898302.6680865, 3644898307.668372, 3644898312.668658, 3644898317.667944, 3644898322.6682296, 3644898327.668516, 3644898332.6678014, 3644898337.668088, 3644898342.6683736, 3644898347.66866, 3644898352.6679454, 3644898357.668232, 3644898362.6685176, 3644898367.667804, 3644898372.6680894, 3644898377.668376, 3644898382.6686616, 3644898387.667948, 3644898392.6682334, 3644898397.66852, 3644898402.6678057, 3644898407.6680913, 3644898412.6683774, 3644898417.668664, 3644898422.6679497], [296.0, 296.1, 295.89, 295.78, 295.94, 295.91, 295.97, 296.12, 296.01, 296.1, 296.01, 296.2, 296.14, 296.06, 296.16, 296.08, 295.89, 295.97, 296.06, 296.03, 296.09, 295.99, 295.89, 295.85, 295.93, 295.74, 295.91, 296.21, 296.04, 296.14, 296.12, 295.91, 296.2, 295.91, 295.87, 296.09, 296.19, 295.91, 296.03, 296.12, 295.94, 296.03, 295.97, 296.01, 296.08, 295.89, 295.91, 295.97, 296.03, 295.81, 295.91, 296.1, 296.15, 296.05, 296.15, 296.24, 295.82, 295.81, 296.14, 296.24, 295.97, 296.06, 295.74, 295.95, 296.08, 295.94, 295.91, 295.91, 296.12]}, {[3644898082.6645026, 3644898087.663789, 3644898092.6640744, 3644898097.66436, 3644898102.6646466, 3644898107.663933, 3644898112.6642184, 3644898117.664504, 3644898122.66379, 3644898127.664076, 3644898132.6643624, 3644898137.665648, 3644898142.6649346, 3644898147.66522, 3644898152.6655064, 3644898157.664792, 3644898162.665078, 3644898167.665364, 3644898172.6656504, 3644898177.664936, 3644898182.665222, 3644898187.665508, 3644898192.6647944, 3644898197.66508, 3644898202.6663666, 3644898207.666652, 3644898212.6659384, 3644898217.666224, 3644898222.6665106, 3644898227.665796, 3644898232.6660824, 3644898237.667368, 3644898242.6676545, 3644898247.66694, 3644898252.6672263, 3644898257.667512, 3644898262.6667986, 3644898267.667084, 3644898272.6673694, 3644898277.667656, 3644898282.6669426, 3644898287.667228, 3644898292.6675134, 3644898297.6678, 3644898302.6680865, 3644898307.668372, 3644898312.668658, 3644898317.667944, 3644898322.6682296, 3644898327.668516, 3644898332.6678014, 3644898337.668088, 3644898342.6683736, 3644898347.66866, 3644898352.6679454, 3644898357.668232, 3644898362.6685176, 3644898367.667804, 3644898372.6680894, 3644898377.668376, 3644898382.6686616, 3644898387.667948, 3644898392.6682334, 3644898397.66852, 3644898402.6678057, 3644898407.6680913, 3644898412.6683774, 3644898417.668664, 3644898422.6679497], [290.48, 291.09, 290.9, 291.1, 290.9, 290.9, 291.04, 291.04, 290.99, 290.93, 290.9, 291.31, 290.97, 291.13, 291.04, 291.12, 290.93, 290.69, 291.06, 291.27, 291.06, 291.04, 290.96, 291.09, 290.86, 290.95, 291.01, 291.18, 291.25, 291.18, 290.95, 291.08, 291.12, 290.97, 290.93, 291.09, 291.27, 291.02, 290.93, 291.08, 291.22, 291.12, 290.92, 290.69, 291.02, 291.02, 290.9, 290.86, 291.08, 290.88, 290.77, 291.01, 291.05, 291.1, 291.14, 290.99, 291.06, 290.9, 291.05, 291.31, 291.05, 291.06, 290.95, 290.99, 290.99, 290.9, 290.9, 290.96, 291.08]}]
  out "U idx":i32[](array[numeric])=[0, 1]
  out "NI DAQ OUT":dbl[](array[numeric])=[-50013.24569663551, 15.025355709698363, -250.03334959533717, -250.04156931728906, -26.29672579614668, -0.7155199244462975, 103537.91205606361, -50000.0, -50000.0] format="%#_3f"
  out "NI-DAQ CH indic.":string[](array[string])=["U1", "U2", "U3", "U4", "U5", "U6", "U7", "U8"]
  out "Graph S. 1":cluster{dbl[], dbl[]}[](graph)
  in  "log/linear 4":bool
  in  "log/linear 1":bool
  out "Graph S. 3":cluster{dbl[], dbl[]}[](graph)
  in  "log/linear 6":bool
  in  "log/linear 3":bool
  in  "log/linear 2":bool
  out "Graph S. 6":cluster{dbl[], dbl[]}[](graph)
  out "Graph S. 5":cluster{dbl[], dbl[]}[](graph)
  in  "log/linear 5":bool
  in  "S.5 SEL":i32[](array[numeric])=[0, 2, 3]
  out "Graph S. 4":cluster{dbl[], dbl[]}[](graph)
  in  "S.1 SEL":i32[](array[numeric])=[0, 2]
  in  "S.2 SEL":i32[](array[numeric])=[1]
  out "Graph S. 2":cluster{dbl[], dbl[]}[](graph)
  in  "S.3 SEL":i32[](array[numeric])=[0, 2, 3]
  in  "S.4 SEL":i32[](array[numeric])=[0, 2, 3]
  in  "S.6 SEL":i32[](array[numeric])=[0, 2, 3]
  in  "DAQ OUT SET Volt":dbl[](array[numeric])=[2.0] format="%0.2f"
  out "DAQ OUT \nsample #":u32=1
  out "Q idx":i32[](array[numeric])=[0, 1]
  out "date/time string":string="20190702_164122_"
  in  "Wait (s)":i32=5
  # "Some time needed until program stops!"
  # "Record Config"
  # "VISA address"
  # "Error states"
  # "CH4 of LSI-D broken!"
  # "NI-DAQ config"
  # "Defines # of measurements \n taken for averaging"
  # "Inputs on this page have to be filled before the start of the program"
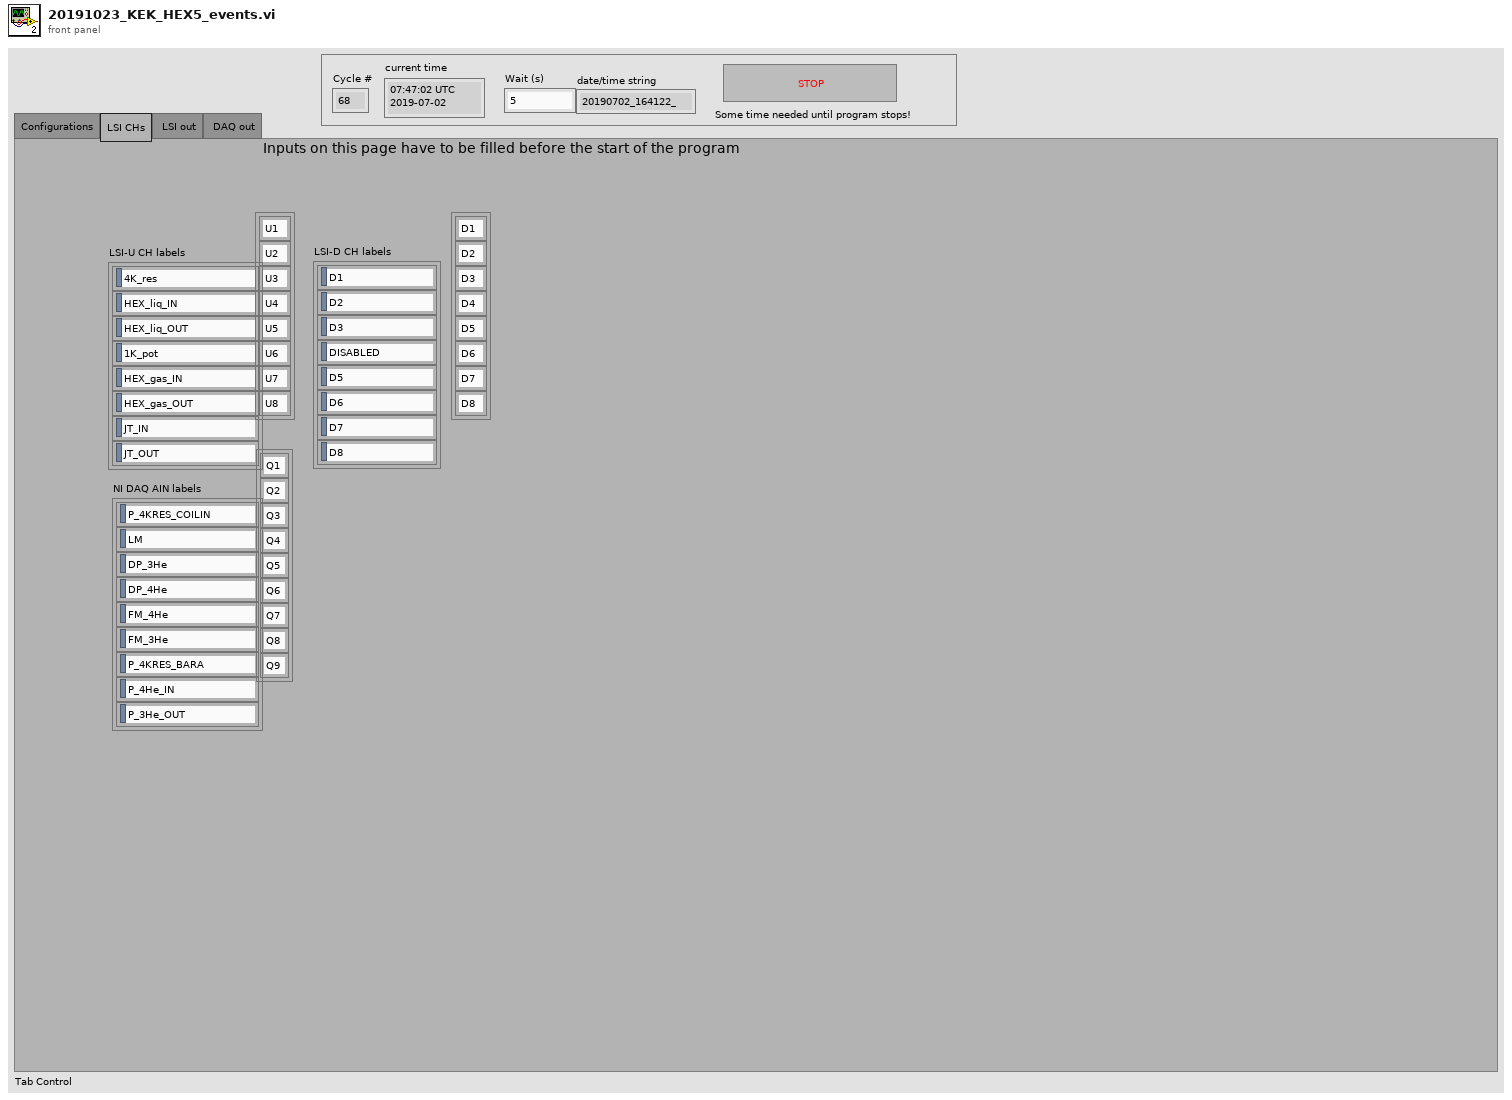
[diagram p1: front panel]
types:
  T1 = enum32{"Configurations", "LSI CHs", " LSI out", " DAQ out"}
  T2 = enum16{"open", "replace", "create", "open or create", "replace or create", "replace or create with confirmation"}
  T3 = cluster{"LSI-U CH labels[0]":string, "LSI-U CH labels[1]":string, "LSI-U CH labels[2]":string, "LSI-U CH labels[3]":string, "LSI-U CH labels[4]":string, "LSI-U CH labels[5]":string, "LSI-U CH labels[6]":string, "LSI-U CH labels[7]":string, "LSI-U CH labels[8]":string}
  T4 = cluster{"LSI-D CH labels[0]":string, "LSI-D CH labels[1]":string, "LSI-D CH labels[2]":string, "LSI-D CH labels[3]":string, "LSI-D CH labels[4]":string, "LSI-D CH labels[5]":string, "LSI-D CH labels[6]":string, "LSI-D CH labels[7]":string, "LSI-D CH labels[8]":string}
  T5 = cluster{"NI DAQ AIN labels[0]":string, "NI DAQ AIN labels[1]":string, "NI DAQ AIN labels[2]":string, "NI DAQ AIN labels[3]":string, "NI DAQ AIN labels[4]":string, "NI DAQ AIN labels[5]":string, "NI DAQ AIN labels[6]":string, "NI DAQ AIN labels[7]":string, "NI DAQ AIN labels[8]":string}
  T6 = cluster{"LSI-D out[0]":dbl, "LSI-D out[1]":dbl, "LSI-D out[2]":dbl, "LSI-D out[3]":dbl, "LSI-D out[4]":dbl, "LSI-D out[5]":dbl, "LSI-D out[6]":dbl, "LSI-D out[7]":dbl, "LSI-D out[8]":dbl}
  T7 = cluster{"LSI-U out[0]":dbl, "LSI-U out[1]":dbl, "LSI-U out[2]":dbl, "LSI-U out[3]":dbl, "LSI-U out[4]":dbl, "LSI-U out[5]":dbl, "LSI-U out[6]":dbl, "LSI-U out[7]":dbl, "LSI-U out[8]":dbl}
  T8 = cluster{"[0]":dbl, "[1]":dbl, "[2]":dbl, "[3]":dbl, "[4]":dbl, "[5]":dbl, "[6]":dbl, "[7]":dbl, "[8]":dbl}
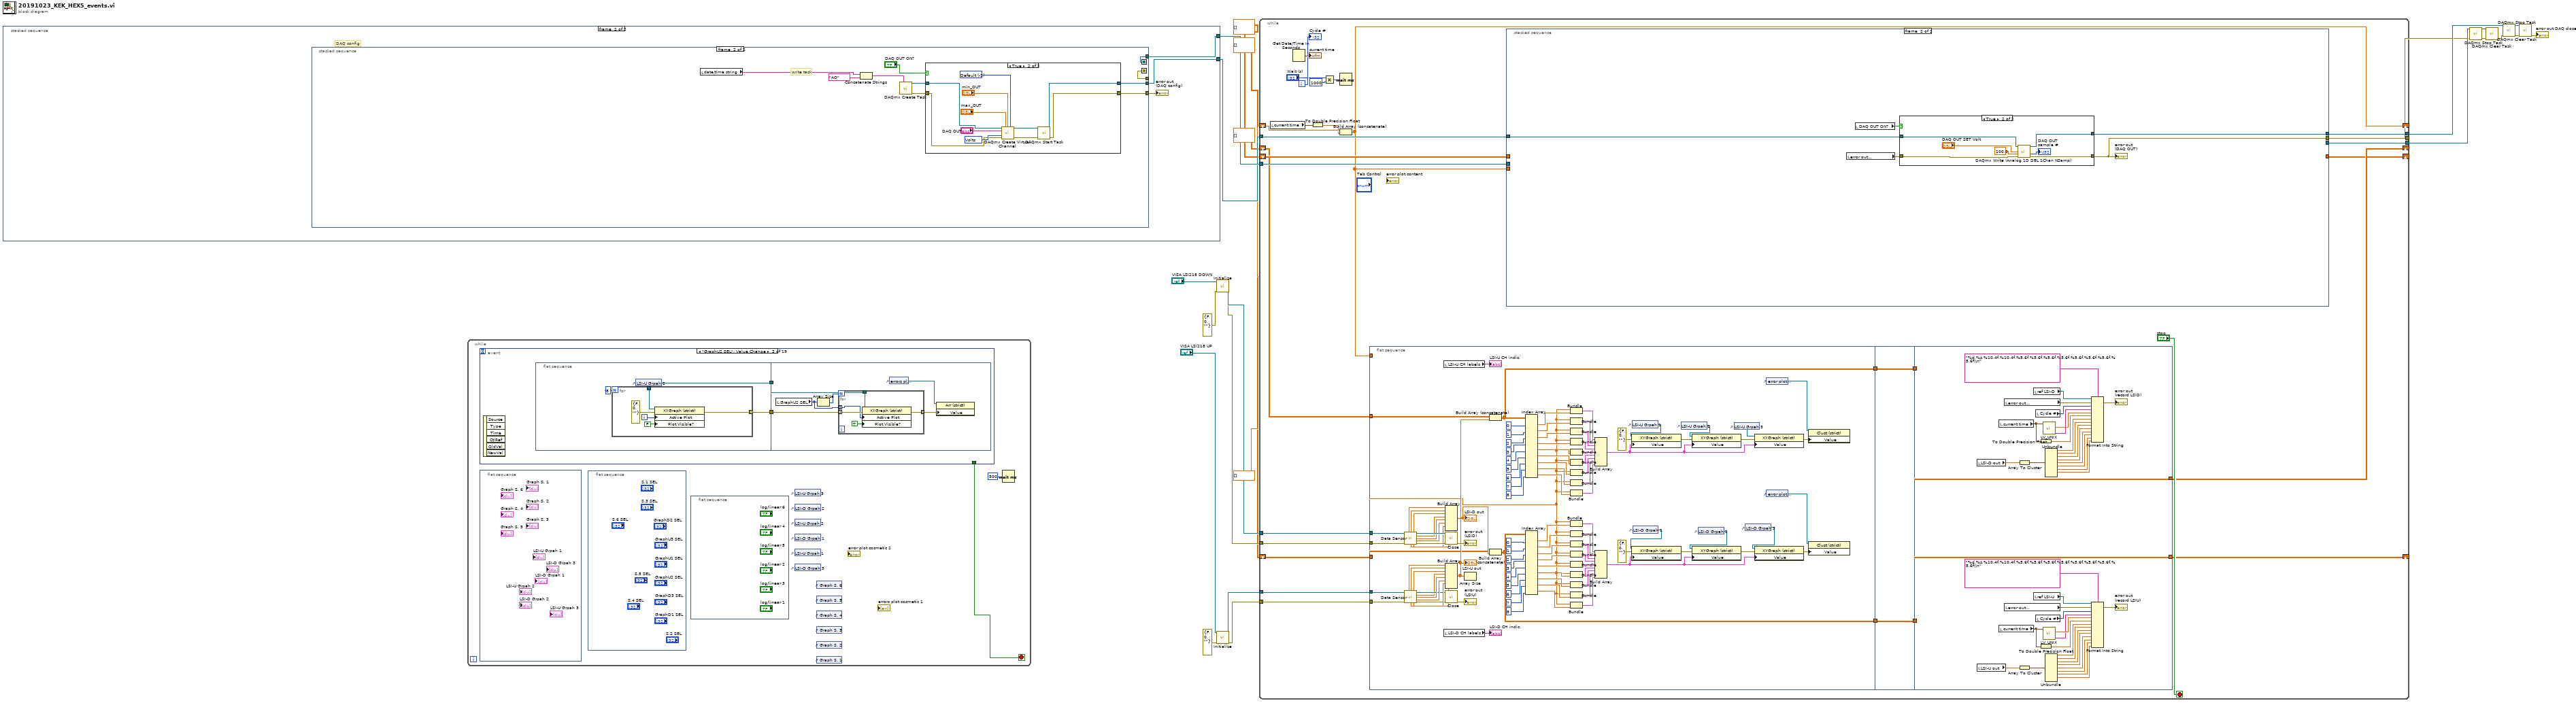
[diagram p0: block diagram]
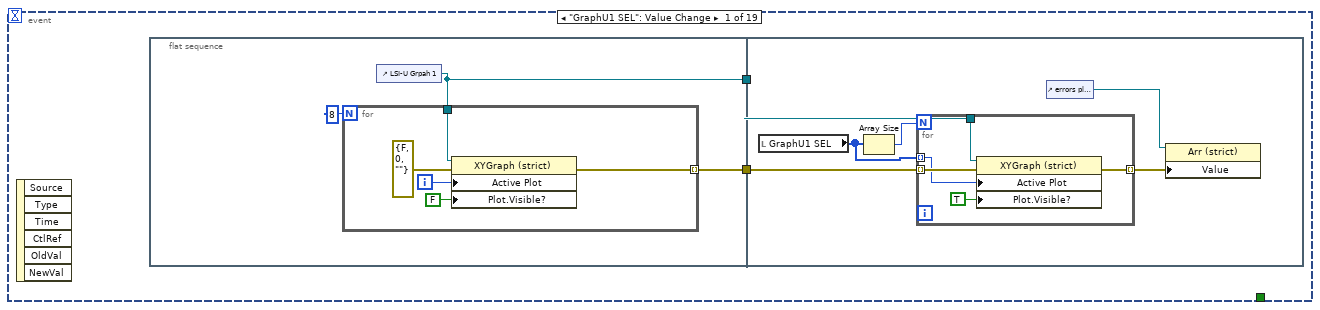
[diagram p2: hidden frame]
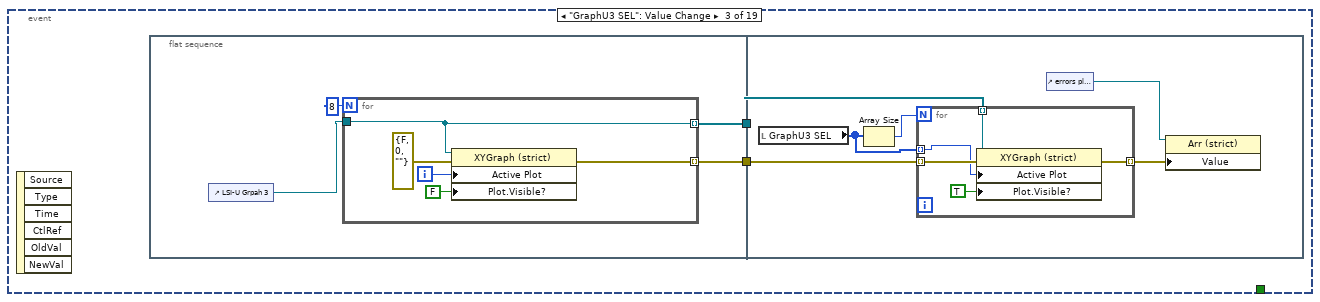
[diagram p3: hidden frame]
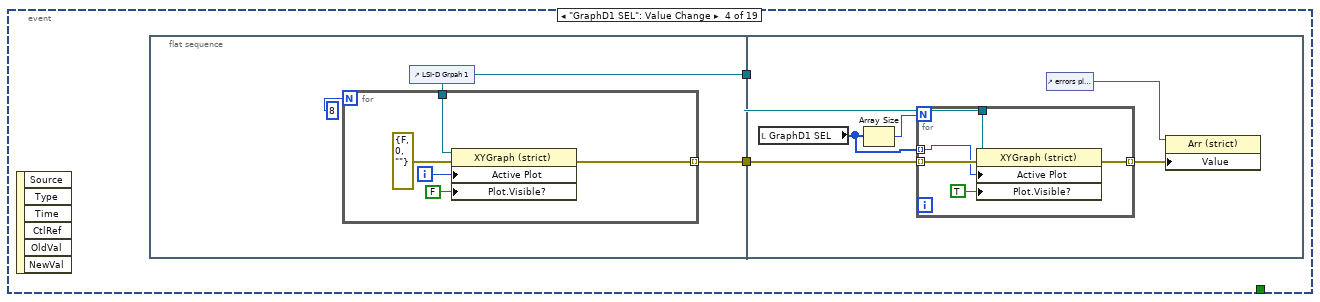
[diagram p4: hidden frame]
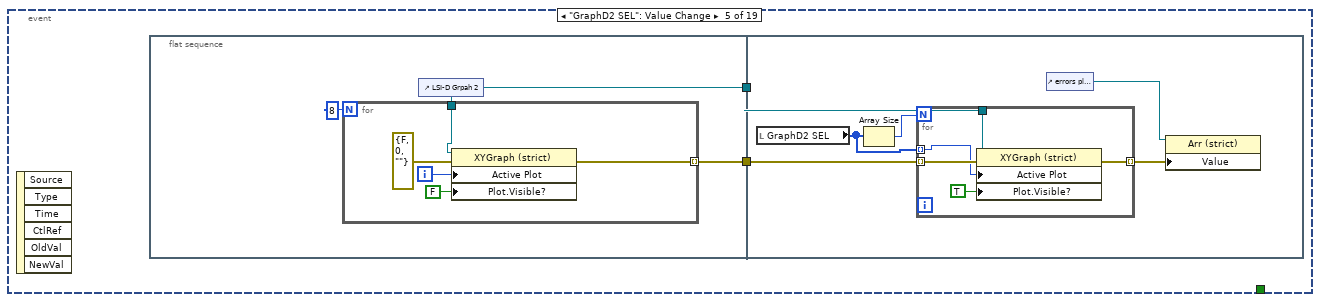
[diagram p5: hidden frame]
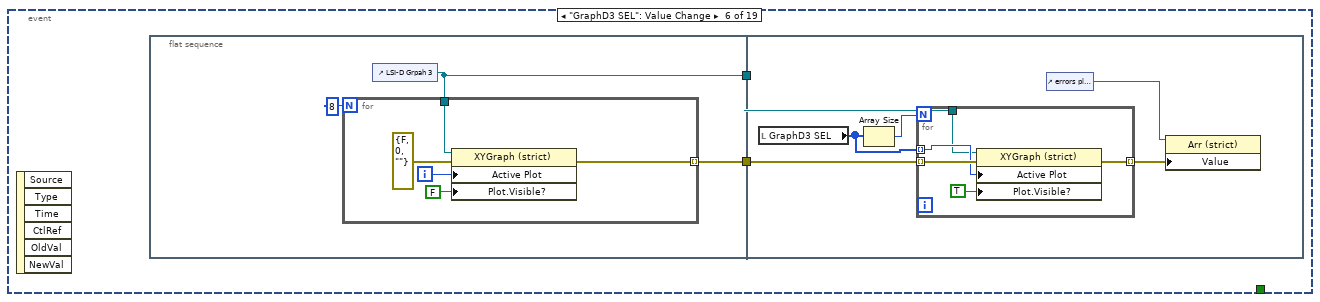
[diagram p6: hidden frame]
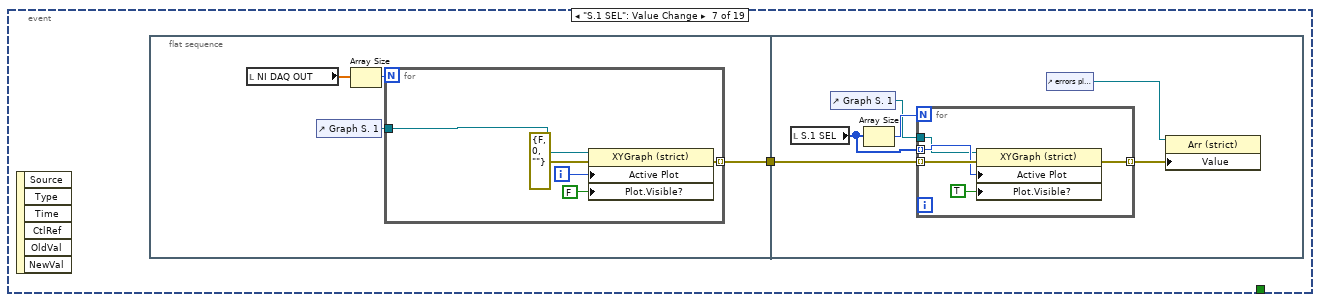
[diagram p7: hidden frame]
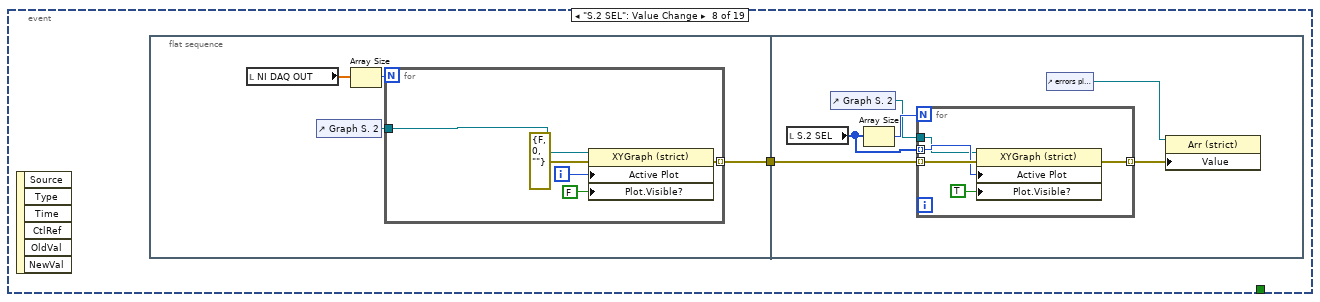
[diagram p8: hidden frame]
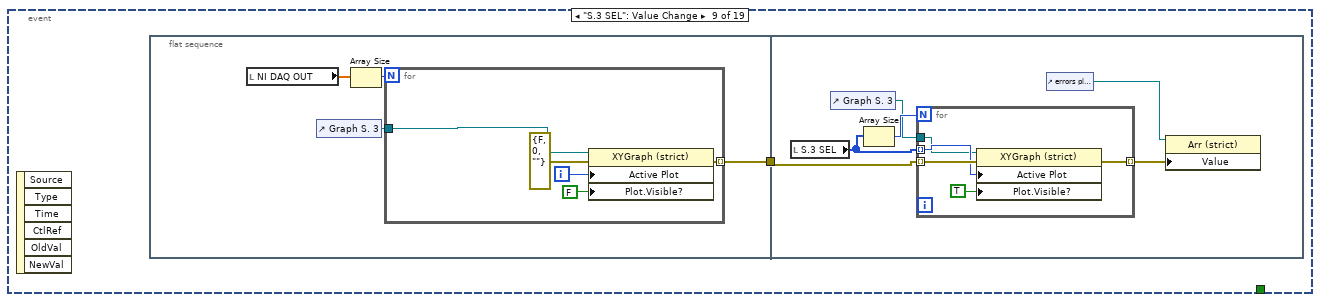
[diagram p9: hidden frame]
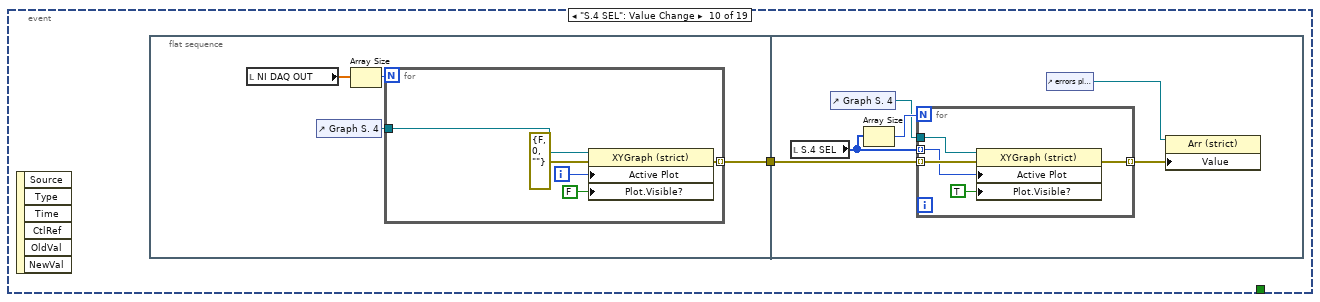
[diagram p10: hidden frame]
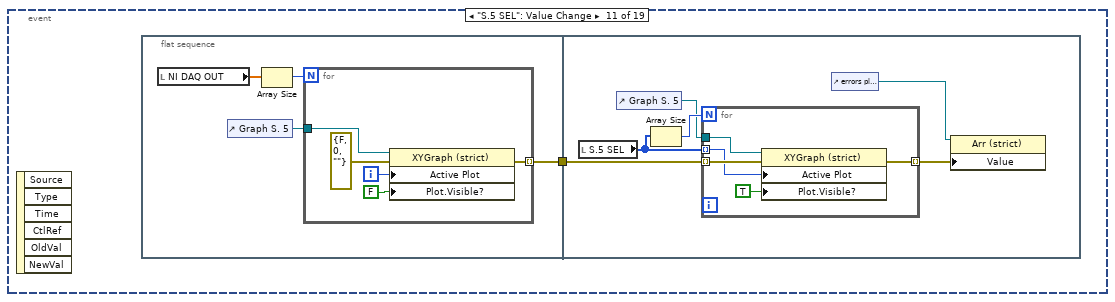
[diagram p11: hidden frame]
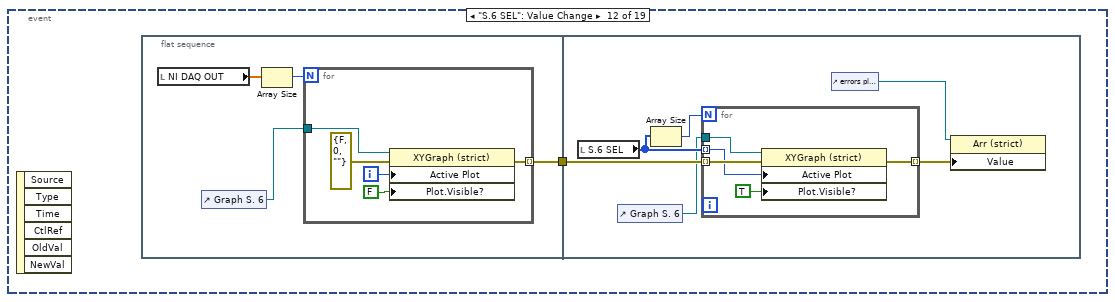
[diagram p12: hidden frame]
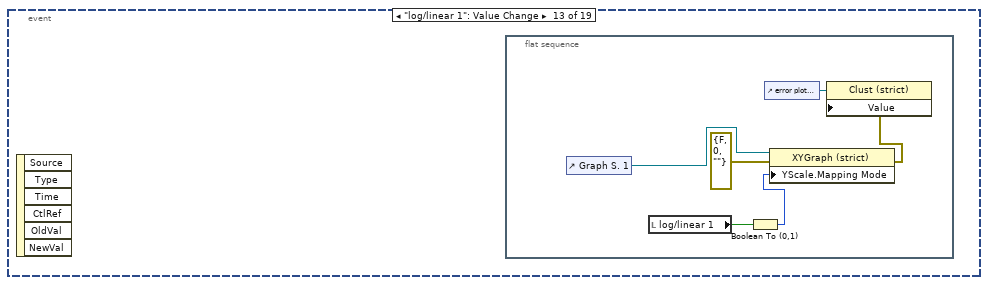
[diagram p13: hidden frame]
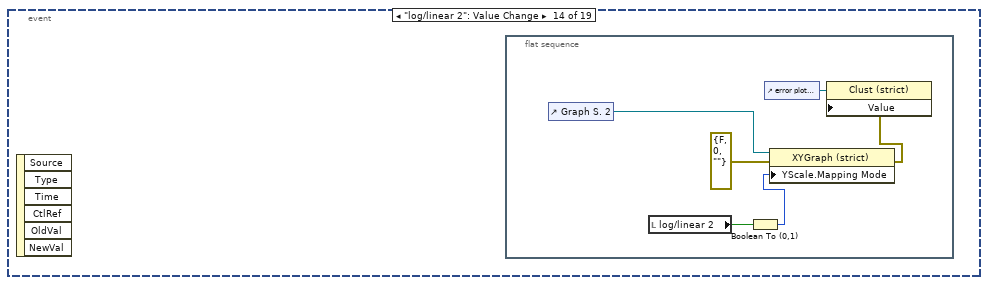
[diagram p14: hidden frame]
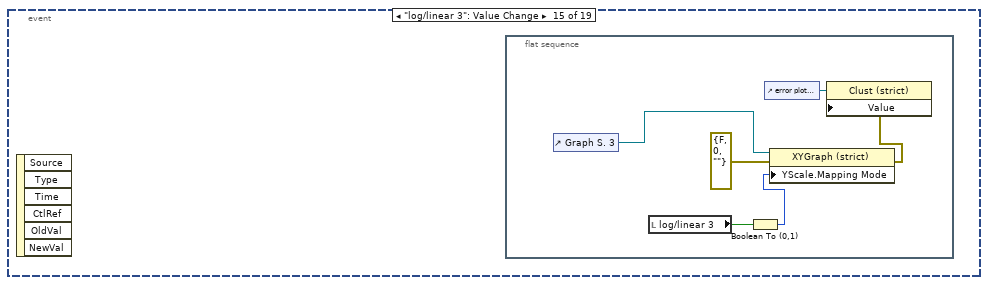
[diagram p15: hidden frame]
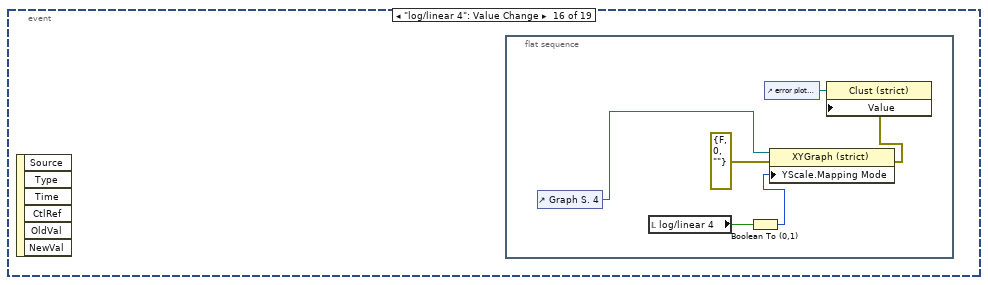
[diagram p16: hidden frame]
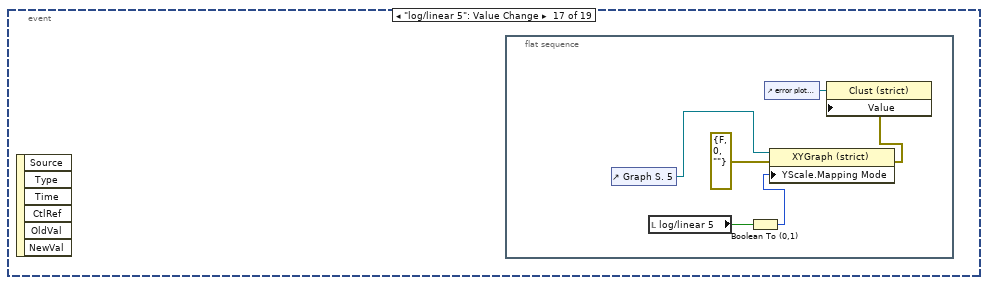
[diagram p17: hidden frame]
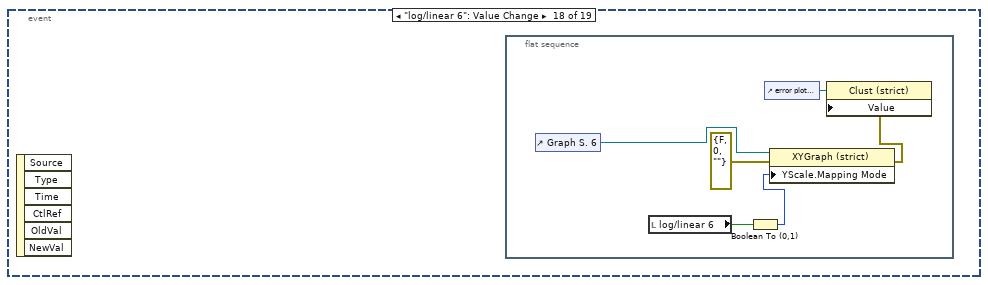
[diagram p18: hidden frame]
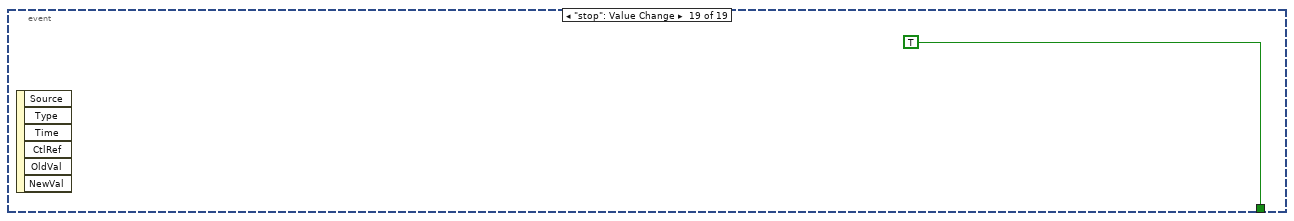
[diagram p19: hidden frame]
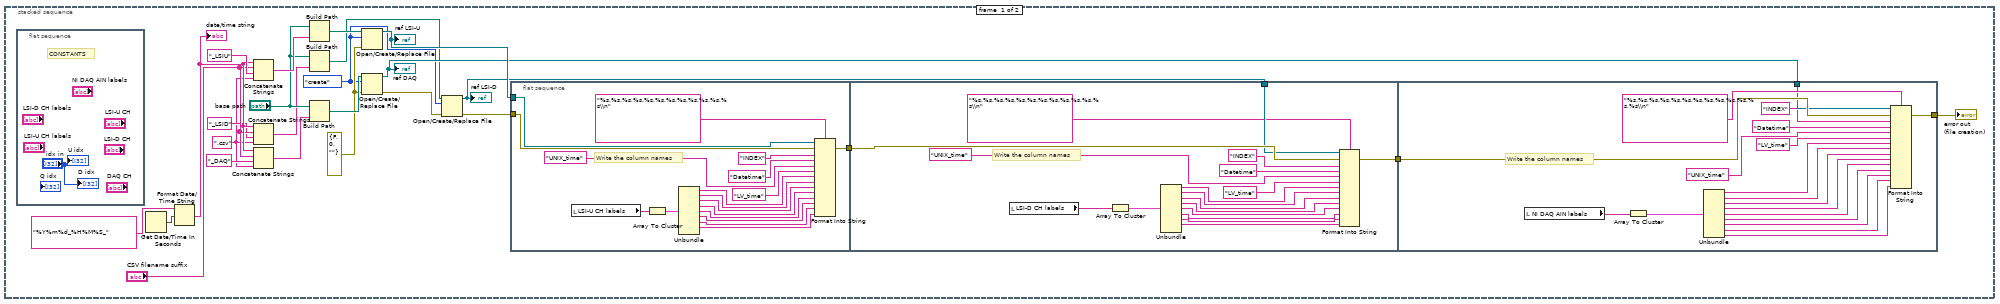
[diagram p20: hidden frame]
diagram:
  n1 = stacked-sequence {
    tunnel: [_ w107] -> w23
    tunnel: [_ w106] -> w22
    frame #0 {
      w40 = errorcluster {"status"=FALSE, "code"=0, "source"=""} ("error in")
      w33 = ".csv" ("string")
      w32 = T2."create" ("operation (0:open)")
      n2 = flat-sequence {
        frame #0 {
          # "CONSTANTS"
          "U idx" <- "idx in"
          "D idx" <- "idx in"
        }
      }
      n3 = Get Date/Time In Seconds() -> (seconds since 1Jan1904=w48:timestamp)
      n4 = Format Date/Time String(time format string (%c)="%Y%m%d_%H%M%S_", seconds (now)=w48) -> (date/time string=w36:string)  [unwired: 1 in]
      "date/time string" <- w36
      n5 = Concatenate Strings(w36, "CSV filename suffix", "_LSIU" ("string"), w33) -> (w45:string)
      n6 = Concatenate Strings(w36, "CSV filename suffix", "_LSID" ("string"), w33) -> (w30:string)
      n7 = Concatenate Strings(w36, "CSV filename suffix", "_DAQ" ("string"), w33) -> (w43:string)
      n8 = Build Path(base path="base path", name or relative path=w45) -> (appended path=w46:path)
      n9 = Build Path(base path="base path", name or relative path=w30) -> (appended path=w29:path)
      n10 = Build Path(base path="base path", name or relative path=w43) -> (appended path=w41:path)
      n11 = Open/Create/Replace File(file path (use dialog)=w46, error in=w40, operation (0:open)=w32) -> (refnum out=w39:refnum<file>)  [unwired: 3 in, 2 out]
      "ref LSI-U" <- w39
      n12 = Open/Create/Replace File(file path (use dialog)=w41, error in=w40, operation (0:open)=w32) -> (refnum out=w38:refnum<file>, error out=w28:errorcluster)  [unwired: 3 in, 1 out]
      "ref DAQ" <- w38
      n13 = Open/Create/Replace File(file path (use dialog)=w29, error in=w28, operation (0:open)=w32) -> (refnum out=w24:refnum<file>, error out=w27:errorcluster)  [unwired: 3 in, 1 out]
      "ref LSI-D" <- w24
      n14 = flat-sequence {
        tunnel: w39 -> [w66]
        tunnel: w27 -> [w65]
        tunnel: [w61] -> w26
        tunnel: w26 -> [w71]
        tunnel: [w70] -> w25
        tunnel: w24 -> [w69]
        tunnel: w25 -> [w100]
        tunnel: w38 -> [w99]
        tunnel: [w98] -> w37
        frame #0 {
          # "Write the column names"
          n15 = local read "LSI-U CH labels"() -> (w59:string[])
          n16 = Array To Cluster(array=w59) -> (cluster=w58:T3)
          n17 = Unbundle(w58) -> ("LSI-U CH labels[0]"=w57:string, "LSI-U CH labels[1]"=w56:string, "LSI-U CH labels[2]"=w55:string, "LSI-U CH labels[3]"=w54:string, "LSI-U CH labels[4]"=w53:string, "LSI-U CH labels[5]"=w52:string, "LSI-U CH labels[6]"=w51:string, "LSI-U CH labels[7]"=w50:string)  [unwired: 1 out]
          n18 = Format Into String(format string="%s,%s,%s,%s,%s,%s,%s,%s,%s,%s,%s,%s\\n" ("time format string (%c)"), initial string=w66, error in=w65, "INDEX" ("input 1"), "Datetime" ("input 1"), "UNIX_time" ("input 1"), "LV_time" ("input 1"), w57, w56, w55, w54, w53, w52, w51, w50) -> (error out=w61:errorcluster)  [unwired: 1 out]
        }
        frame #1 {
          # "Write the column names"
          n19 = local read "LSI-D CH labels"() -> (w76:string[])
          n20 = Array To Cluster(array=w76) -> (cluster=w77:T4)
          n21 = Unbundle(w77) -> ("LSI-D CH labels[0]"=w78:string, "LSI-D CH labels[1]"=w79:string, "LSI-D CH labels[2]"=w80:string, "LSI-D CH labels[3]"=w81:string, "LSI-D CH labels[4]"=w82:string, "LSI-D CH labels[5]"=w83:string, "LSI-D CH labels[6]"=w84:string, "LSI-D CH labels[7]"=w85:string)  [unwired: 1 out]
          n22 = Format Into String(format string="%s,%s,%s,%s,%s,%s,%s,%s,%s,%s,%s,%s\\n" ("time format string (%c)"), initial string=w69, error in=w71, "INDEX" ("input 1"), "Datetime" ("input 1"), "UNIX_time" ("input 1"), "LV_time" ("input 1"), w78, w79, w80, w81, w82, w83, w84, w85) -> (error out=w70:errorcluster)  [unwired: 1 out]
        }
        frame #2 {
          # "Write the column names"
          n23 = local read "NI DAQ AIN labels"() -> (w96:string[])
          n24 = Array To Cluster(array=w96) -> (cluster=w95:T5)
          n25 = Unbundle(w95) -> ("NI DAQ AIN labels[0]"=w94:string, "NI DAQ AIN labels[1]"=w93:string, "NI DAQ AIN labels[2]"=w92:string, "NI DAQ AIN labels[3]"=w91:string, "NI DAQ AIN labels[4]"=w90:string, "NI DAQ AIN labels[5]"=w89:string, "NI DAQ AIN labels[6]"=w88:string, "NI DAQ AIN labels[7]"=w87:string, "NI DAQ AIN labels[8]"=w86:string)
          n26 = Format Into String(format string="%s,%s,%s,%s,%s,%s,%s,%s,%s,%s,%s,%s,%s\\n" ("time format string (%c)"), initial string=w99, error in=w100, "INDEX" ("input 1"), "Datetime" ("input 1"), "UNIX_time" ("input 1"), "LV_time" ("input 1"), w94, w93, w92, w91, w90, w89, w88, w87, w86) -> (error out=w98:errorcluster)  [unwired: 1 out]
        }
      }
      "error out\n(file creation)" <- w37
    }
    frame #1 {
      # "DAQ config"
      n27 = stacked-sequence {
        seq-local: [w156 _] -> [_ w171]
        seq-local: [w155 _] -> [_ w170]
        tunnel: [_ w171] -> _
        tunnel: [_ w170] -> w107
        tunnel: [_ w169] -> w106
        tunnel: [_ w168] -> w105
        frame #0 {
          w108 = 10106 items=["Default"=-1, "RSE"=10083, "NRSE"=10078, "Differential"=10106, "Pseudodifferential"=12529] ("input terminal configuration")
          # "read task"
          n28 = local read "date/time string"() -> (w128:string)
          n29 = Concatenate Strings(w128, "AI" ("new task name")) -> (w126:string)
          n30 = call <vilib>:"DAQmx Create Task.vi"("new task name"=w126, "error in"=errorcluster {"status"=FALSE, "code"=0, "source"=""}) -> ("task out"=w157:refnum<k21>, "error out"=w159:errorcluster)  [unwired: 12 in]
          n31 = call-poly <vilib>:"DAQmx Create Virtual Channel.vi"("task in"=w157, "maximum value"="max_P", "minimum value"="min_P", "input terminal configuration"=w108, "physical channels"="DAQ IN: P (4He coil out)", "error in"=w159) -> ("task out"=w149:refnum<k21>, "error out"=w158:errorcluster)  [unwired: 8 in]
          n32 = call-poly <vilib>:"DAQmx Create Virtual Channel.vi"("task in"=w149, "maximum value"="max_LM", "minimum value"="min_LM", "input terminal configuration"=w108, "physical channels"="DAQ IN: He-level", "error in"=w158) -> ("task out"=w146:refnum<k21>, "error out"=w139:errorcluster)  [unwired: 8 in]
          n33 = call-poly <vilib>:"DAQmx Create Virtual Channel.vi"("task in"=w146, "maximum value"="max_dP4", "minimum value"="min_dP4", "input terminal configuration"=w108, "physical channels"="DAQ IN: ƒ¢P (4He)", "error in"=w139) -> ("task out"=w152:refnum<k21>, "error out"=w151:errorcluster)  [unwired: 8 in]
          n34 = call-poly <vilib>:"DAQmx Create Virtual Channel.vi"("task in"=w152, "maximum value"="max_dP3", "minimum value"="min_dP3", "input terminal configuration"=w108, "physical channels"="DAQ IN: ƒ¢P (3He)", "error in"=w151) -> ("task out"=w141:refnum<k21>, "error out"=w138:errorcluster)  [unwired: 8 in]
          n35 = call-poly <vilib>:"DAQmx Create Virtual Channel.vi"("task in"=w141, "maximum value"="max_FM4", "minimum value"="min_FM4", "input terminal configuration"=w108, "physical channels"="DAQ IN: FM (4He)", "error in"=w138) -> ("task out"=w133:refnum<k21>, "error out"=w131:errorcluster)  [unwired: 8 in]
          n36 = call-poly <vilib>:"DAQmx Create Virtual Channel.vi"("task in"=w133, "maximum value"="max_FM3", "minimum value"="min_FM3", "input terminal configuration"=w108, "physical channels"="DAQ IN: FM (3He)", "error in"=w131) -> ("task out"=w124:refnum<k21>, "error out"=w125:errorcluster)  [unwired: 8 in]
          n37 = call-poly <vilib>:"DAQmx Create Virtual Channel.vi"("task in"=w124, "maximum value"="max_BARA", "minimum value"="min_BARA", "input terminal configuration"=w108, "physical channels"="DAQ IN: BARA", "error in"=w125) -> ("task out"=w120:refnum<k21>, "error out"=w119:errorcluster)  [unwired: 8 in]
          n38 = call-poly <vilib>:"DAQmx Create Virtual Channel.vi"("task in"=w120, "maximum value"="max_P4HeIN", "minimum value"="min_P4HeIN", "input terminal configuration"=w108, "physical channels"="DAQ IN: P_4HeIN", "error in"=w119) -> ("task out"=w111:refnum<k21>, "error out"=w113:errorcluster)  [unwired: 8 in]
          n39 = call-poly <vilib>:"DAQmx Create Virtual Channel.vi"("task in"=w111, "maximum value"="max_P3HeOUT", "minimum value"="min_P3HeOUT", "input terminal configuration"=w108, "physical channels"="DAQ IN: P_3HeOUT", "error in"=w113) -> ("task out"=w115:refnum<k21>, "error out"=w114:errorcluster)  [unwired: 8 in]
          n40 = call <vilib>:"DAQmx Start Task.vi"("task/channels in"=w115, "error in"=w114) -> ("task out"=w155:refnum<k21>, "error out"=w156:errorcluster)  [unwired: 12 in]
        }
        frame #1 {
          # "write task"
          n41 = local read "date/time string"() -> (w164:string)
          n42 = Concatenate Strings(w164, "AO" ("new task name")) -> (w162:string)
          n43 = call <vilib>:"DAQmx Create Task.vi"("new task name"=w162) -> ("task out"=w166:refnum<k21>, "error out"=w165:errorcluster)  [unwired: 13 in]
          n44 = case shown="True" "DAQ OUT ON?" {
            tunnel: [w173 w180] -> w169
            tunnel: [w172 w179] -> w168
            tunnel: w166 -> [w173 w178]
            tunnel: w165 -> [w172 w177]
            frame False {
            }
            frame True {
              w182 = -1 items=["Default"=-1, "RSE"=10083, "Differential"=10106, "Pseudodifferential"=12529] ("output terminal configuration")
              w181 = 10348 items=["Volts"=10348, "From Custom Scale"=10065] ("units")
              n45 = call-poly <vilib>:"DAQmx Create Virtual Channel.vi"("task in"=w178, "maximum value"="max_OUT", "minimum value"="min_OUT", "output terminal configuration"=w182, "physical channels"="DAQ OUT", "units"=w181, "error in"=w177) -> ("task out"=w184:refnum<k21>, "error out"=w183:errorcluster)  [unwired: 7 in]
              n46 = call <vilib>:"DAQmx Start Task.vi"("task/channels in"=w184, "error in"=w183) -> ("task out"=w180:refnum<k21>, "error out"=w179:errorcluster)  [unwired: 12 in]
            }
          }
        }
      }
      "error out\n(DAQ config)" <- w105
    }
  }
  n47 = while {
    stop <- w185 stop-if-true
    n48 = event shown="[1] \"GraphU2 SEL\": Value Change" {
      selector: _ -> [_ _ _ _ _ _ _ _ _ _ _ _ _ _ _ _ _ _ _]
      dyn-events: _ -> [_ _ _ _ _ _ _ _ _ _ _ _ _ _ _ _ _ _ _]
      timeout: _ -> [_ _ _ _ _ _ _ _ _ _ _ _ _ _ _ _ _ _ _]
      tunnel: [_ _ _ _ _ _ _ _ _ _ _ _ _ _ _ _ _ _ TRUE] -> w185
      event "GraphU1 SEL": Value Change {
        n49 = event-data() -> ()  [unwired: 1 in, 6 out]
        n50 = flat-sequence {
          tunnel: [w191] -> w188
          tunnel: [w189] -> w187
          tunnel: w188 -> [w200]
          tunnel: w187 -> [w197]
          frame #0 {
            n51 = control-ref of="LSI-U Grpah 1"() -> (w189:refnum<vi>)
            n52 = for {
              N: 8 -> [_]
              tunnel: [w193] -> w191 mode=indexing
              tunnel: w189 -> [w192]
              i -> [w195]
              n53 = property class="XYGraph (strict)"(reference=w192, error in=errorcluster {"status"=FALSE, "code"=0, "source"=""} ("error in (no error)"), "Active Plot"=w195, "Plot.Visible?"=FALSE ("Plot.Visible")) -> (error out=w193:errorcluster)  [unwired: 1 out]
            }
          }
          frame #1 {
            n54 = local read "GraphU1 SEL"() -> (w201:i32[])
            n55 = Array Size(array=w201) -> (size(s)=w202:i32)
            n56 = for {
              N: w202 -> [_]
              tunnel: w201 -> [w206] mode=indexing
              tunnel: w200 -> [w207] mode=indexing
              tunnel: [w204] -> w198 mode=indexing
              tunnel: w197 -> [w203]
              n57 = property class="XYGraph (strict)"(reference=w203, error in=w207, "Active Plot"=w206, "Plot.Visible?"=TRUE ("Plot.Visible")) -> (error out=w204:errorcluster)  [unwired: 1 out]
            }
            n58 = control-ref of="errors plot cosmetic 1"() -> (w199:refnum<vi>)
            n59 = property class="Arr (strict)"(reference=w199, "Value"=w198) -> ()  [unwired: 1 in, 2 out]
          }
        }
      }
      event "GraphU2 SEL": Value Change {
        n60 = event-data() -> ()  [unwired: 1 in, 6 out]
        n61 = flat-sequence {
          tunnel: [w212] -> w209
          tunnel: [w210] -> w208
          tunnel: w209 -> [w221]
          tunnel: w208 -> [w218]
          frame #0 {
            n62 = control-ref of="LSI-U Grpah 2"() -> (w210:refnum<vi>)
            n63 = for {
              N: 8 -> [_]
              tunnel: [w214] -> w212 mode=indexing
              tunnel: w210 -> [w213]
              i -> [w216]
              n64 = property class="XYGraph (strict)"(reference=w213, error in=errorcluster {"status"=FALSE, "code"=0, "source"=""} ("error in (no error)"), "Active Plot"=w216, "Plot.Visible?"=FALSE ("Plot.Visible")) -> (error out=w214:errorcluster)  [unwired: 1 out]
            }
          }
          frame #1 {
            n65 = local read "GraphU2 SEL"() -> (w222:i32[])
            n66 = Array Size(array=w222) -> (size(s)=w223:i32)
            n67 = for {
              N: w223 -> [_]
              tunnel: w222 -> [w227] mode=indexing
              tunnel: w221 -> [w228] mode=indexing
              tunnel: [w225] -> w219 mode=indexing
              tunnel: w218 -> [w224]
              n68 = property class="XYGraph (strict)"(reference=w224, error in=w228, "Active Plot"=w227, "Plot.Visible?"=TRUE ("Plot.Visible")) -> (error out=w225:errorcluster)  [unwired: 1 out]
            }
            n69 = control-ref of="errors plot cosmetic 1"() -> (w220:refnum<vi>)
            n70 = property class="Arr (strict)"(reference=w220, "Value"=w219) -> ()  [unwired: 1 in, 2 out]
          }
        }
      }
      event "GraphU3 SEL": Value Change {
        n71 = event-data() -> ()  [unwired: 1 in, 6 out]
        n72 = flat-sequence {
          tunnel: [w234] -> w230
          tunnel: [w231] -> w229
          tunnel: w230 -> [w243]
          tunnel: w229 -> [w240]
          frame #0 {
            n73 = control-ref of="LSI-U Grpah 3"() -> (w232:refnum<vi>)
            n74 = for {
              N: 8 -> [_]
              tunnel: [w236] -> w234 mode=indexing
              tunnel: w232 -> [w235]
              tunnel: [w235] -> w231 mode=indexing
              i -> [w238]
              n75 = property class="XYGraph (strict)"(reference=w235, error in=errorcluster {"status"=FALSE, "code"=0, "source"=""} ("error in (no error)"), "Active Plot"=w238, "Plot.Visible?"=FALSE ("Plot.Visible")) -> (error out=w236:errorcluster)  [unwired: 1 out]
            }
          }
          frame #1 {
            n76 = local read "GraphU3 SEL"() -> (w244:i32[])
            n77 = Array Size(array=w244) -> (size(s)=w245:i32)
            n78 = for {
              N: w245 -> [_]
              tunnel: w244 -> [w249] mode=indexing
              tunnel: w243 -> [w250] mode=indexing
              tunnel: [w247] -> w241 mode=indexing
              tunnel: w240 -> [w246] mode=indexing
              n79 = property class="XYGraph (strict)"(reference=w246, error in=w250, "Active Plot"=w249, "Plot.Visible?"=TRUE ("Plot.Visible")) -> (error out=w247:errorcluster)  [unwired: 1 out]
            }
            n80 = control-ref of="errors plot cosmetic 1"() -> (w242:refnum<vi>)
            n81 = property class="Arr (strict)"(reference=w242, "Value"=w241) -> ()  [unwired: 1 in, 2 out]
          }
        }
      }
      event "GraphD1 SEL": Value Change {
        n82 = event-data() -> ()  [unwired: 1 in, 6 out]
        n83 = flat-sequence {
          tunnel: [w255] -> w252
          tunnel: [w253] -> w251
          tunnel: w252 -> [w264]
          tunnel: w251 -> [w261]
          frame #0 {
            n84 = control-ref of="LSI-D Grpah 1"() -> (w253:refnum<vi>)
            n85 = for {
              N: 8 -> [_]
              tunnel: [w257] -> w255 mode=indexing
              tunnel: w253 -> [w256]
              i -> [w259]
              n86 = property class="XYGraph (strict)"(reference=w256, error in=errorcluster {"status"=FALSE, "code"=0, "source"=""} ("error in (no error)"), "Active Plot"=w259, "Plot.Visible?"=FALSE ("Plot.Visible")) -> (error out=w257:errorcluster)  [unwired: 1 out]
            }
          }
          frame #1 {
            n87 = local read "GraphD1 SEL"() -> (w265:i32[])
            n88 = Array Size(array=w265) -> (size(s)=w266:i32)
            n89 = for {
              N: w266 -> [_]
              tunnel: w265 -> [w270] mode=indexing
              tunnel: w264 -> [w271] mode=indexing
              tunnel: [w268] -> w262 mode=indexing
              tunnel: w261 -> [w267]
              n90 = property class="XYGraph (strict)"(reference=w267, error in=w271, "Active Plot"=w270, "Plot.Visible?"=TRUE ("Plot.Visible")) -> (error out=w268:errorcluster)  [unwired: 1 out]
            }
            n91 = control-ref of="errors plot cosmetic 1"() -> (w263:refnum<vi>)
            n92 = property class="Arr (strict)"(reference=w263, "Value"=w262) -> ()  [unwired: 1 in, 2 out]
          }
        }
      }
      event "GraphD2 SEL": Value Change {
        n93 = event-data() -> ()  [unwired: 1 in, 6 out]
        n94 = flat-sequence {
          tunnel: [w276] -> w273
          tunnel: [w274] -> w272
          tunnel: w273 -> [w285]
          tunnel: w272 -> [w282]
          frame #0 {
            n95 = control-ref of="LSI-D Grpah 2"() -> (w274:refnum<vi>)
            n96 = for {
              N: 8 -> [_]
              tunnel: [w278] -> w276 mode=indexing
              tunnel: w274 -> [w277]
              i -> [w280]
              n97 = property class="XYGraph (strict)"(reference=w277, error in=errorcluster {"status"=FALSE, "code"=0, "source"=""} ("error in (no error)"), "Active Plot"=w280, "Plot.Visible?"=FALSE ("Plot.Visible")) -> (error out=w278:errorcluster)  [unwired: 1 out]
            }
          }
          frame #1 {
            n98 = local read "GraphD2 SEL"() -> (w286:i32[])
            n99 = Array Size(array=w286) -> (size(s)=w287:i32)
            n100 = for {
              N: w287 -> [_]
              tunnel: w286 -> [w291] mode=indexing
              tunnel: w285 -> [w292] mode=indexing
              tunnel: [w289] -> w283 mode=indexing
              tunnel: w282 -> [w288]
              n101 = property class="XYGraph (strict)"(reference=w288, error in=w292, "Active Plot"=w291, "Plot.Visible?"=TRUE ("Plot.Visible")) -> (error out=w289:errorcluster)  [unwired: 1 out]
            }
            n102 = control-ref of="errors plot cosmetic 1"() -> (w284:refnum<vi>)
            n103 = property class="Arr (strict)"(reference=w284, "Value"=w283) -> ()  [unwired: 1 in, 2 out]
          }
        }
      }
      event "GraphD3 SEL": Value Change {
        n104 = event-data() -> ()  [unwired: 1 in, 6 out]
        n105 = flat-sequence {
          tunnel: [w297] -> w294
          tunnel: [w295] -> w293
          tunnel: w294 -> [w306]
          tunnel: w293 -> [w303]
          frame #0 {
            n106 = control-ref of="LSI-D Grpah 3"() -> (w295:refnum<vi>)
            n107 = for {
              N: 8 -> [_]
              tunnel: [w299] -> w297 mode=indexing
              tunnel: w295 -> [w298]
              i -> [w301]
              n108 = property class="XYGraph (strict)"(reference=w298, error in=errorcluster {"status"=FALSE, "code"=0, "source"=""} ("error in (no error)"), "Active Plot"=w301, "Plot.Visible?"=FALSE ("Plot.Visible")) -> (error out=w299:errorcluster)  [unwired: 1 out]
            }
          }
          frame #1 {
            n109 = local read "GraphD3 SEL"() -> (w307:i32[])
            n110 = Array Size(array=w307) -> (size(s)=w308:i32)
            n111 = for {
              N: w308 -> [_]
              tunnel: w307 -> [w312] mode=indexing
              tunnel: w306 -> [w313] mode=indexing
              tunnel: [w310] -> w304 mode=indexing
              tunnel: w303 -> [w309]
              n112 = property class="XYGraph (strict)"(reference=w309, error in=w313, "Active Plot"=w312, "Plot.Visible?"=TRUE ("Plot.Visible")) -> (error out=w310:errorcluster)  [unwired: 1 out]
            }
            n113 = control-ref of="errors plot cosmetic 1"() -> (w305:refnum<vi>)
            n114 = property class="Arr (strict)"(reference=w305, "Value"=w304) -> ()  [unwired: 1 in, 2 out]
          }
        }
      }
      event "S.1 SEL": Value Change {
        n115 = event-data() -> ()  [unwired: 1 in, 6 out]
        n116 = flat-sequence {
          tunnel: [w318] -> w314
          tunnel: w314 -> [w327]
          frame #0 {
            n117 = local read "NI DAQ OUT"() -> (w316:dbl[])
            n118 = control-ref of="Graph S. 1"() -> (w317:refnum<vi>)
            n119 = Array Size(array=w316) -> (size(s)=w315:i32)
            n120 = for {
              N: w315 -> [_]
              tunnel: [w320] -> w318 mode=indexing
              tunnel: w317 -> [w319]
              i -> [w322]
              n121 = property class="XYGraph (strict)"(reference=w319, error in=errorcluster {"status"=FALSE, "code"=0, "source"=""} ("error in (no error)"), "Active Plot"=w322, "Plot.Visible?"=FALSE ("Plot.Visible")) -> (error out=w320:errorcluster)  [unwired: 1 out]
            }
          }
          frame #1 {
            n122 = local read "S.1 SEL"() -> (w328:i32[])
            n123 = control-ref of="Graph S. 1"() -> (w324:refnum<vi>)
            n124 = Array Size(array=w328) -> (size(s)=w329:i32)
            n125 = for {
              N: w329 -> [_]
              tunnel: w328 -> [w333] mode=indexing
              tunnel: w327 -> [w334] mode=indexing
              tunnel: [w331] -> w325 mode=indexing
              tunnel: w324 -> [w330]
              n126 = property class="XYGraph (strict)"(reference=w330, error in=w334, "Active Plot"=w333, "Plot.Visible?"=TRUE ("Plot.Visible")) -> (error out=w331:errorcluster)  [unwired: 1 out]
            }
            n127 = control-ref of="errors plot cosmetic 1"() -> (w326:refnum<vi>)
            n128 = property class="Arr (strict)"(reference=w326, "Value"=w325) -> ()  [unwired: 1 in, 2 out]
          }
        }
      }
      event "S.2 SEL": Value Change {
        n129 = event-data() -> ()  [unwired: 1 in, 6 out]
        n130 = flat-sequence {
          tunnel: [w339] -> w335
          tunnel: w335 -> [w348]
          frame #0 {
            n131 = local read "NI DAQ OUT"() -> (w338:dbl[])
            n132 = control-ref of="Graph S. 2"() -> (w336:refnum<vi>)
            n133 = Array Size(array=w338) -> (size(s)=w337:i32)
            n134 = for {
              N: w337 -> [_]
              tunnel: [w341] -> w339 mode=indexing
              tunnel: w336 -> [w340]
              i -> [w343]
              n135 = property class="XYGraph (strict)"(reference=w340, error in=errorcluster {"status"=FALSE, "code"=0, "source"=""} ("error in (no error)"), "Active Plot"=w343, "Plot.Visible?"=FALSE ("Plot.Visible")) -> (error out=w341:errorcluster)  [unwired: 1 out]
            }
          }
          frame #1 {
            n136 = local read "S.2 SEL"() -> (w349:i32[])
            n137 = control-ref of="Graph S. 2"() -> (w345:refnum<vi>)
            n138 = Array Size(array=w349) -> (size(s)=w350:i32)
            n139 = for {
              N: w350 -> [_]
              tunnel: w349 -> [w354] mode=indexing
              tunnel: w348 -> [w355] mode=indexing
              tunnel: [w352] -> w346 mode=indexing
              tunnel: w345 -> [w351]
              n140 = property class="XYGraph (strict)"(reference=w351, error in=w355, "Active Plot"=w354, "Plot.Visible?"=TRUE ("Plot.Visible")) -> (error out=w352:errorcluster)  [unwired: 1 out]
            }
            n141 = control-ref of="errors plot cosmetic 1"() -> (w347:refnum<vi>)
            n142 = property class="Arr (strict)"(reference=w347, "Value"=w346) -> ()  [unwired: 1 in, 2 out]
          }
        }
      }
      event "S.3 SEL": Value Change {
        n143 = event-data() -> ()  [unwired: 1 in, 6 out]
        n144 = flat-sequence {
          tunnel: [w360] -> w356
          tunnel: w356 -> [w369]
          frame #0 {
            n145 = local read "NI DAQ OUT"() -> (w359:dbl[])
            n146 = control-ref of="Graph S. 3"() -> (w357:refnum<vi>)
            n147 = Array Size(array=w359) -> (size(s)=w358:i32)
            n148 = for {
              N: w358 -> [_]
              tunnel: [w362] -> w360 mode=indexing
              tunnel: w357 -> [w361]
              i -> [w364]
              n149 = property class="XYGraph (strict)"(reference=w361, error in=errorcluster {"status"=FALSE, "code"=0, "source"=""} ("error in (no error)"), "Active Plot"=w364, "Plot.Visible?"=FALSE ("Plot.Visible")) -> (error out=w362:errorcluster)  [unwired: 1 out]
            }
          }
          frame #1 {
            n150 = local read "S.3 SEL"() -> (w370:i32[])
            n151 = control-ref of="Graph S. 3"() -> (w366:refnum<vi>)
            n152 = Array Size(array=w370) -> (size(s)=w371:i32)
            n153 = for {
              N: w371 -> [_]
              tunnel: w370 -> [w375] mode=indexing
              tunnel: w369 -> [w376] mode=indexing
              tunnel: [w373] -> w367 mode=indexing
              tunnel: w366 -> [w372]
              n154 = property class="XYGraph (strict)"(reference=w372, error in=w376, "Active Plot"=w375, "Plot.Visible?"=TRUE ("Plot.Visible")) -> (error out=w373:errorcluster)  [unwired: 1 out]
            }
            n155 = control-ref of="errors plot cosmetic 1"() -> (w368:refnum<vi>)
            n156 = property class="Arr (strict)"(reference=w368, "Value"=w367) -> ()  [unwired: 1 in, 2 out]
          }
        }
      }
      event "S.4 SEL": Value Change {
        n157 = event-data() -> ()  [unwired: 1 in, 6 out]
        n158 = flat-sequence {
          tunnel: [w381] -> w377
          tunnel: w377 -> [w390]
          frame #0 {
            n159 = local read "NI DAQ OUT"() -> (w380:dbl[])
            n160 = control-ref of="Graph S. 4"() -> (w378:refnum<vi>)
            n161 = Array Size(array=w380) -> (size(s)=w379:i32)
            n162 = for {
              N: w379 -> [_]
              tunnel: [w383] -> w381 mode=indexing
              tunnel: w378 -> [w382]
              i -> [w385]
              n163 = property class="XYGraph (strict)"(reference=w382, error in=errorcluster {"status"=FALSE, "code"=0, "source"=""} ("error in (no error)"), "Active Plot"=w385, "Plot.Visible?"=FALSE ("Plot.Visible")) -> (error out=w383:errorcluster)  [unwired: 1 out]
            }
          }
          frame #1 {
            n164 = local read "S.4 SEL"() -> (w391:i32[])
            n165 = control-ref of="Graph S. 4"() -> (w387:refnum<vi>)
            n166 = Array Size(array=w391) -> (size(s)=w392:i32)
            n167 = for {
              N: w392 -> [_]
              tunnel: w391 -> [w396] mode=indexing
              tunnel: w390 -> [w397] mode=indexing
              tunnel: [w394] -> w388 mode=indexing
              tunnel: w387 -> [w393]
              n168 = property class="XYGraph (strict)"(reference=w393, error in=w397, "Active Plot"=w396, "Plot.Visible?"=TRUE ("Plot.Visible")) -> (error out=w394:errorcluster)  [unwired: 1 out]
            }
            n169 = control-ref of="errors plot cosmetic 1"() -> (w389:refnum<vi>)
            n170 = property class="Arr (strict)"(reference=w389, "Value"=w388) -> ()  [unwired: 1 in, 2 out]
          }
        }
      }
      event "S.5 SEL": Value Change {
        n171 = event-data() -> ()  [unwired: 1 in, 6 out]
        n172 = flat-sequence {
          tunnel: [w402] -> w398
          tunnel: w398 -> [w411]
          frame #0 {
            n173 = local read "NI DAQ OUT"() -> (w401:dbl[])
            n174 = control-ref of="Graph S. 5"() -> (w399:refnum<vi>)
            n175 = Array Size(array=w401) -> (size(s)=w400:i32)
            n176 = for {
              N: w400 -> [_]
              tunnel: [w404] -> w402 mode=indexing
              tunnel: w399 -> [w403]
              i -> [w406]
              n177 = property class="XYGraph (strict)"(reference=w403, error in=errorcluster {"status"=FALSE, "code"=0, "source"=""} ("error in (no error)"), "Active Plot"=w406, "Plot.Visible?"=FALSE ("Plot.Visible")) -> (error out=w404:errorcluster)  [unwired: 1 out]
            }
          }
          frame #1 {
            n178 = local read "S.5 SEL"() -> (w412:i32[])
            n179 = control-ref of="Graph S. 5"() -> (w408:refnum<vi>)
            n180 = Array Size(array=w412) -> (size(s)=w413:i32)
            n181 = for {
              N: w413 -> [_]
              tunnel: w412 -> [w417] mode=indexing
              tunnel: w411 -> [w418] mode=indexing
              tunnel: [w415] -> w409 mode=indexing
              tunnel: w408 -> [w414]
              n182 = property class="XYGraph (strict)"(reference=w414, error in=w418, "Active Plot"=w417, "Plot.Visible?"=TRUE ("Plot.Visible")) -> (error out=w415:errorcluster)  [unwired: 1 out]
            }
            n183 = control-ref of="errors plot cosmetic 1"() -> (w410:refnum<vi>)
            n184 = property class="Arr (strict)"(reference=w410, "Value"=w409) -> ()  [unwired: 1 in, 2 out]
          }
        }
      }
      event "S.6 SEL": Value Change {
        n185 = event-data() -> ()  [unwired: 1 in, 6 out]
        n186 = flat-sequence {
          tunnel: [w423] -> w419
          tunnel: w419 -> [w432]
          frame #0 {
            n187 = local read "NI DAQ OUT"() -> (w422:dbl[])
            n188 = control-ref of="Graph S. 6"() -> (w420:refnum<vi>)
            n189 = Array Size(array=w422) -> (size(s)=w421:i32)
            n190 = for {
              N: w421 -> [_]
              tunnel: [w425] -> w423 mode=indexing
              tunnel: w420 -> [w424]
              i -> [w427]
              n191 = property class="XYGraph (strict)"(reference=w424, error in=errorcluster {"status"=FALSE, "code"=0, "source"=""} ("error in (no error)"), "Active Plot"=w427, "Plot.Visible?"=FALSE ("Plot.Visible")) -> (error out=w425:errorcluster)  [unwired: 1 out]
            }
          }
          frame #1 {
            n192 = local read "S.6 SEL"() -> (w433:i32[])
            n193 = control-ref of="Graph S. 6"() -> (w429:refnum<vi>)
            n194 = Array Size(array=w433) -> (size(s)=w434:i32)
            n195 = for {
              N: w434 -> [_]
              tunnel: w433 -> [w438] mode=indexing
              tunnel: w432 -> [w439] mode=indexing
              tunnel: [w436] -> w430 mode=indexing
              tunnel: w429 -> [w435]
              n196 = property class="XYGraph (strict)"(reference=w435, error in=w439, "Active Plot"=w438, "Plot.Visible?"=TRUE ("Plot.Visible")) -> (error out=w436:errorcluster)  [unwired: 1 out]
            }
            n197 = control-ref of="errors plot cosmetic 1"() -> (w431:refnum<vi>)
            n198 = property class="Arr (strict)"(reference=w431, "Value"=w430) -> ()  [unwired: 1 in, 2 out]
          }
        }
      }
      event "log/linear 1": Value Change {
        n199 = event-data() -> ()  [unwired: 1 in, 6 out]
        n200 = flat-sequence {
          frame #0 {
            n201 = control-ref of="Graph S. 1"() -> (w444:refnum<vi>)
            n202 = local read "log/linear 1"() -> (w443:bool)
            n203 = Boolean To (0,1)(Boolean=w443) -> (0, 1=w442:i16)
            n204 = control-ref of="error plot cosmetic 2"() -> (w441:refnum<vi>)
            n205 = property class="XYGraph (strict)"(reference=w444, error in=errorcluster {"status"=FALSE, "code"=0, "source"=""} ("error in (no error)"), "YScale.Mapping Mode"=w442) -> (error out=w440:errorcluster)  [unwired: 1 out]
            n206 = property class="Clust (strict)"(reference=w441, "Value"=w440) -> ()  [unwired: 1 in, 2 out]
          }
        }
      }
      event "log/linear 2": Value Change {
        n207 = event-data() -> ()  [unwired: 1 in, 6 out]
        n208 = flat-sequence {
          frame #0 {
            n209 = control-ref of="Graph S. 2"() -> (w446:refnum<vi>)
            n210 = local read "log/linear 2"() -> (w450:bool)
            n211 = Boolean To (0,1)(Boolean=w450) -> (0, 1=w449:i16)
            n212 = control-ref of="error plot cosmetic 2"() -> (w448:refnum<vi>)
            n213 = property class="XYGraph (strict)"(reference=w446, error in=errorcluster {"status"=FALSE, "code"=0, "source"=""} ("error in (no error)"), "YScale.Mapping Mode"=w449) -> (error out=w447:errorcluster)  [unwired: 1 out]
            n214 = property class="Clust (strict)"(reference=w448, "Value"=w447) -> ()  [unwired: 1 in, 2 out]
          }
        }
      }
      event "log/linear 3": Value Change {
        n215 = event-data() -> ()  [unwired: 1 in, 6 out]
        n216 = flat-sequence {
          frame #0 {
            n217 = control-ref of="Graph S. 3"() -> (w452:refnum<vi>)
            n218 = local read "log/linear 3"() -> (w456:bool)
            n219 = Boolean To (0,1)(Boolean=w456) -> (0, 1=w455:i16)
            n220 = control-ref of="error plot cosmetic 2"() -> (w454:refnum<vi>)
            n221 = property class="XYGraph (strict)"(reference=w452, error in=errorcluster {"status"=FALSE, "code"=0, "source"=""} ("error in (no error)"), "YScale.Mapping Mode"=w455) -> (error out=w453:errorcluster)  [unwired: 1 out]
            n222 = property class="Clust (strict)"(reference=w454, "Value"=w453) -> ()  [unwired: 1 in, 2 out]
          }
        }
      }
      event "log/linear 4": Value Change {
        n223 = event-data() -> ()  [unwired: 1 in, 6 out]
        n224 = flat-sequence {
          frame #0 {
            n225 = control-ref of="Graph S. 4"() -> (w458:refnum<vi>)
            n226 = local read "log/linear 4"() -> (w462:bool)
            n227 = Boolean To (0,1)(Boolean=w462) -> (0, 1=w461:i16)
            n228 = control-ref of="error plot cosmetic 2"() -> (w460:refnum<vi>)
            n229 = property class="XYGraph (strict)"(reference=w458, error in=errorcluster {"status"=FALSE, "code"=0, "source"=""} ("error in (no error)"), "YScale.Mapping Mode"=w461) -> (error out=w459:errorcluster)  [unwired: 1 out]
            n230 = property class="Clust (strict)"(reference=w460, "Value"=w459) -> ()  [unwired: 1 in, 2 out]
          }
        }
      }
      event "log/linear 5": Value Change {
        n231 = event-data() -> ()  [unwired: 1 in, 6 out]
        n232 = flat-sequence {
          frame #0 {
            n233 = control-ref of="Graph S. 5"() -> (w464:refnum<vi>)
            n234 = local read "log/linear 5"() -> (w468:bool)
            n235 = Boolean To (0,1)(Boolean=w468) -> (0, 1=w467:i16)
            n236 = control-ref of="error plot cosmetic 2"() -> (w466:refnum<vi>)
            n237 = property class="XYGraph (strict)"(reference=w464, error in=errorcluster {"status"=FALSE, "code"=0, "source"=""} ("error in (no error)"), "YScale.Mapping Mode"=w467) -> (error out=w465:errorcluster)  [unwired: 1 out]
            n238 = property class="Clust (strict)"(reference=w466, "Value"=w465) -> ()  [unwired: 1 in, 2 out]
          }
        }
      }
      event "log/linear 6": Value Change {
        n239 = event-data() -> ()  [unwired: 1 in, 6 out]
        n240 = flat-sequence {
          frame #0 {
            n241 = control-ref of="Graph S. 6"() -> (w470:refnum<vi>)
            n242 = local read "log/linear 6"() -> (w474:bool)
            n243 = Boolean To (0,1)(Boolean=w474) -> (0, 1=w473:i16)
            n244 = control-ref of="error plot cosmetic 2"() -> (w472:refnum<vi>)
            n245 = property class="XYGraph (strict)"(reference=w470, error in=errorcluster {"status"=FALSE, "code"=0, "source"=""} ("error in (no error)"), "YScale.Mapping Mode"=w473) -> (error out=w471:errorcluster)  [unwired: 1 out]
            n246 = property class="Clust (strict)"(reference=w472, "Value"=w471) -> ()  [unwired: 1 in, 2 out]
          }
        }
      }
      event "stop": Value Change {
        n247 = event-data() -> ()  [unwired: 1 in, 6 out]
      }
    }
    n248 = flat-sequence {
      frame #0 {
      }
    }
    n249 = flat-sequence {
      frame #0 {
      }
    }
    n250 = flat-sequence {
      frame #0 {
      }
    }
    n251 = control-ref of="LSI-U Grpah 3"() -> ()  [unwired: 1 out]
    n252 = control-ref of="LSI-D Grpah 2"() -> ()  [unwired: 1 out]
    n253 = control-ref of="LSI-U Grpah 2"() -> ()  [unwired: 1 out]
    n254 = control-ref of="LSI-D Grpah 1"() -> ()  [unwired: 1 out]
    n255 = control-ref of="LSI-U Grpah 1"() -> ()  [unwired: 1 out]
    n256 = control-ref of="LSI-D Grpah 3"() -> ()  [unwired: 1 out]
    n257 = control-ref of="Graph S. 6"() -> ()  [unwired: 1 out]
    n258 = control-ref of="Graph S. 5"() -> ()  [unwired: 1 out]
    n259 = control-ref of="Graph S. 4"() -> ()  [unwired: 1 out]
    n260 = control-ref of="Graph S. 3"() -> ()  [unwired: 1 out]
    n261 = control-ref of="Graph S. 2"() -> ()  [unwired: 1 out]
    n262 = control-ref of="Graph S. 1"() -> ()  [unwired: 1 out]
    n263 = Wait (ms)(milliseconds to wait=u32 500) -> ()  [unwired: 1 out]
  }
  n264 = call "Initialize.vi"("VISA resource name"="VISA LSI218 DOWN", "error in (no error)"=errorcluster {"status"=FALSE, "code"=0, "source"=""}) -> ("VISA resource name out"=w6:refnum<visa-resource-name>, "error out"=w5:errorcluster)  [unwired: 12 in]
  n265 = call "Initialize.vi"("VISA resource name"="VISA LSI218 UP", "error in (no error)"=errorcluster {"status"=FALSE, "code"=0, "source"=""}) -> ("VISA resource name out"=w4:refnum<visa-resource-name>, "error out"=w3:errorcluster)  [unwired: 12 in]
  n266 = while {
    shift-right: [w492] -> _
    shift-left: dbl[] [] -> [w503]
    shift-right: [w495] -> _
    shift-left: dbl[][] [] -> [w496]
    tunnel: w23 -> [w499]
    tunnel: w22 -> [w498]
    shift-right: [w491] -> _
    shift-left: dbl[][] [] -> [w497]
    tunnel: [w487] -> w12
    tunnel: [w486] -> w11
    tunnel: [w485] -> w10
    tunnel: w6 -> [w484]
    tunnel: w5 -> [w483]
    tunnel: w4 -> [w482]
    tunnel: w3 -> [w481]
    shift-right: [w478] -> _
    shift-left: dbl[][] [] -> [w477]
    i -> [w500]
    stop <- "stop" stop-if-true
    n267 = local read "current time"() -> (w501:timestamp)
    n268 = Get Date/Time In Seconds() -> (seconds since 1Jan1904=→"current time":timestamp)
    n269 = To Double Precision Float(number=w501) -> (double precision float=w502:dbl)
    n270 = Multiply(x="Wait (s)", y=1000) -> (x*y=w488:i32)
    n271 = Wait (ms)(milliseconds to wait=w488) -> ()  [unwired: 1 out]
    n272 = Build Array (concatenate)(w503, w502) -> (w492:dbl[])
    n273 = flat-sequence {
      tunnel: w492 -> [w731]
      tunnel: w496 -> [w809]
      tunnel: [w798] -> w493
      tunnel: w484 -> [w805]
      tunnel: w483 -> [w804]
      tunnel: w482 -> [w803]
      tunnel: w481 -> [w802]
      tunnel: [w732] -> w479
      tunnel: w477 -> [w733]
      tunnel: [w821] -> w494
      tunnel: w493 -> [w821]
      tunnel: [w820] -> w480
      tunnel: w479 -> [w820]
      tunnel: [w846] -> w495
      tunnel: w494 -> [w846]
      tunnel: [w841] -> w478
      tunnel: w480 -> [w841]
      frame #0 {
        n274 = call "Data Sensor.vi"("VISA resource name"=w805, "error in (no error)"=w804) -> ("Input 1"=w770:dbl, "Input 2"=w769:dbl, "Input 3"=w768:dbl, "VISA resource name out"=w807:refnum<visa-resource-name>, "Input 4"=w767:dbl, "Input 5"=w766:dbl, "Input 6"=w765:dbl, "Input 8"=w763:dbl, "Input 7"=w764:dbl, "error out"=w806:errorcluster)  [unwired: 4 in]
        n275 = call "Data Sensor.vi"("VISA resource name"=w803, "error in (no error)"=w802) -> ("Input 1"=w819:dbl, "Input 2"=w818:dbl, "Input 3"=w817:dbl, "VISA resource name out"=w811:refnum<visa-resource-name>, "Input 4"=w801:dbl, "Input 5"=w816:dbl, "Input 6"=w815:dbl, "Input 8"=w813:dbl, "Input 7"=w814:dbl, "error out"=w812:errorcluster)  [unwired: 4 in]
        n276 = local read "LSI-U CH labels"() -> (→"LSI-U CH indic,":string[])
        n277 = local read "LSI-D CH labels"() -> (→"LSI-D CH indic.":string[])
        n278 = Build Array(w770, w769, w768, w767, w766, w765, w764, w763) -> (w734:dbl[])
        "LSI-D out" <- w734
        n279 = call "Close.vi"("VISA resource name"=w807, "error in (no error)"=w806) -> ("error out"=→"error out \n(LSID)":errorcluster)  [unwired: 13 in]
        n280 = Build Array(w819, w818, w817, w801, w816, w815, w814, w813) -> (w799:dbl[])
        "LSI-U out" <- w799
        n281 = call "Close.vi"("VISA resource name"=w811, "error in (no error)"=w812) -> ("error out"=→"error out \n(LSIU)":errorcluster)  [unwired: 13 in]
        n282 = Array Size(array=w799) -> ()  [unwired: 1 out]
        n283 = Build Array (concatenate)(w809, w799) -> (w798:dbl[][])
        n284 = Build Array (concatenate)(w733, w734) -> (w732:dbl[][])
        n285 = Index Array(array=w798, index (col) #1=0 ("disabled index (col)"), index (col) #2=1 ("index (col)"), index (col) #3=2 ("index (col)"), index (col) #4=3 ("index (col)"), index (col) #5=4 ("index (col)"), index (col) #6=5 ("index (col)"), index (col) #7=6 ("index (col)"), index (col) #8=7 ("index (col)"), index (col) #9=8 ("index (col)")) -> (element #1=w796:dbl[], element #2=w787:dbl[], element #3=w786:dbl[], element #4=w785:dbl[], element #5=w784:dbl[], element #6=w783:dbl[], element #7=w782:dbl[], element #8=w781:dbl[], element #9=w780:dbl[])  [unwired: 9 in]
        n286 = Index Array(array=w732, index (col) #1=0 ("disabled index (col)"), index (col) #2=1 ("index (col)"), index (col) #3=2 ("index (col)"), index (col) #4=3 ("index (col)"), index (col) #5=4 ("index (col)"), index (col) #6=5 ("index (col)"), index (col) #7=6 ("index (col)"), index (col) #8=7 ("index (col)"), index (col) #9=8 ("index (col)")) -> (element #1=w736:dbl[], element #2=w745:dbl[], element #3=w746:dbl[], element #4=w747:dbl[], element #5=w748:dbl[], element #6=w749:dbl[], element #7=w750:dbl[], element #8=w751:dbl[], element #9=w752:dbl[])  [unwired: 9 in]
        n287 = Bundle(w731, w796) -> (w779:cluster{dbl[], dbl[]})  [unwired: 1 in]
        n288 = Bundle(w731, w787) -> (w778:cluster{dbl[], dbl[]})  [unwired: 1 in]
        n289 = Bundle(w731, w786) -> (w777:cluster{dbl[], dbl[]})  [unwired: 1 in]
        n290 = Bundle(w731, w785) -> (w776:cluster{dbl[], dbl[]})  [unwired: 1 in]
        n291 = Bundle(w731, w784) -> (w775:cluster{dbl[], dbl[]})  [unwired: 1 in]
        n292 = Bundle(w731, w783) -> (w774:cluster{dbl[], dbl[]})  [unwired: 1 in]
        n293 = Bundle(w731, w782) -> (w773:cluster{dbl[], dbl[]})  [unwired: 1 in]
        n294 = Bundle(w731, w781) -> (w772:cluster{dbl[], dbl[]})  [unwired: 1 in]
        n295 = Bundle(w731, w780) -> (w771:cluster{dbl[], dbl[]})  [unwired: 1 in]
        n296 = Bundle(w731, w736) -> (w753:cluster{dbl[], dbl[]})  [unwired: 1 in]
        n297 = Bundle(w731, w745) -> (w754:cluster{dbl[], dbl[]})  [unwired: 1 in]
        n298 = Bundle(w731, w746) -> (w755:cluster{dbl[], dbl[]})  [unwired: 1 in]
        n299 = Bundle(w731, w747) -> (w756:cluster{dbl[], dbl[]})  [unwired: 1 in]
        n300 = Bundle(w731, w748) -> (w757:cluster{dbl[], dbl[]})  [unwired: 1 in]
        n301 = Bundle(w731, w749) -> (w758:cluster{dbl[], dbl[]})  [unwired: 1 in]
        n302 = Bundle(w731, w750) -> (w759:cluster{dbl[], dbl[]})  [unwired: 1 in]
        n303 = Bundle(w731, w751) -> (w760:cluster{dbl[], dbl[]})  [unwired: 1 in]
        n304 = Bundle(w731, w752) -> (w761:cluster{dbl[], dbl[]})  [unwired: 1 in]
        n305 = Build Array(w779, w778, w777, w776, w775, w774, w773, w772, w771) -> (w730:cluster{dbl[], dbl[]}[])
        n306 = Build Array(w753, w754, w755, w756, w757, w758, w759, w760, w761) -> (w726:cluster{dbl[], dbl[]}[])
        n307 = control-ref of="LSI-U Grpah 1"() -> (w715:refnum<vi>)
        n308 = property class="XYGraph (strict)"(reference=w715, error in=errorcluster {"status"=FALSE, "code"=0, "source"=""} ("error in (no error)"), "Value"=w730) -> (error out=w728:errorcluster)  [unwired: 1 out]
        n309 = control-ref of="LSI-D Grpah 1"() -> (w718:refnum<vi>)
        n310 = property class="XYGraph (strict)"(reference=w718, error in=errorcluster {"status"=FALSE, "code"=0, "source"=""} ("error in (no error)"), "Value"=w726) -> (error out=w724:errorcluster)  [unwired: 1 out]
        n311 = control-ref of="LSI-U Grpah 2"() -> (w714:refnum<vi>)
        n312 = property class="XYGraph (strict)"(reference=w714, error in=w728, "Value"=w730) -> (error out=w727:errorcluster)  [unwired: 1 out]
        n313 = control-ref of="LSI-D Grpah 2"() -> (w717:refnum<vi>)
        n314 = property class="XYGraph (strict)"(reference=w717, error in=w724, "Value"=w726) -> (error out=w723:errorcluster)  [unwired: 1 out]
        n315 = control-ref of="LSI-U Grpah 3"() -> (w713:refnum<vi>)
        n316 = control-ref of="LSI-D Grpah 3"() -> (w716:refnum<vi>)
        n317 = property class="XYGraph (strict)"(reference=w713, error in=w727, "Value"=w730) -> (error out=w719:errorcluster)  [unwired: 1 out]
        n318 = property class="XYGraph (strict)"(reference=w716, error in=w723, "Value"=w726) -> (error out=w721:errorcluster)  [unwired: 1 out]
        n319 = control-ref of="error plot content"() -> (w720:refnum<vi>)
        n320 = control-ref of="error plot content"() -> (w722:refnum<vi>)
        n321 = property class="Clust (strict)"(reference=w720, "Value"=w719) -> ()  [unwired: 1 in, 2 out]
        n322 = property class="Clust (strict)"(reference=w722, "Value"=w721) -> ()  [unwired: 1 in, 2 out]
      }
      frame #1 {
      }
      frame #2 {
        n323 = local read "LSI-D out"() -> (w822:dbl[])
        n324 = local read "LSI-U out"() -> (w857:dbl[])
        n325 = local read "current time"() -> (w837:timestamp)
        n326 = local read "current time"() -> (w845:timestamp)
        n327 = local read "error out\n(file creation)"() -> (w824:errorcluster)
        n328 = local read "error out\n(file creation)"() -> (w860:errorcluster)
        n329 = Array To Cluster(array=w822) -> (cluster=w827:T6)
        n330 = Array To Cluster(array=w857) -> (cluster=w856:T7)
        n331 = local read "ref LSI-D"() -> (w823:refnum<file>)
        n332 = local read "ref LSI-U"() -> (w861:refnum<file>)
        n333 = local read "Cycle #"() -> (w840:i32)
        n334 = local read "Cycle #"() -> (w842:i32)
        n335 = To Double Precision Float(number=w837) -> (double precision float=w825:dbl)
        n336 = To Double Precision Float(number=w845) -> (double precision float=w859:dbl)
        n337 = call "LV_UNIX.vi"("current time"=w837) -> ("date/time string"=w839:string, "UNIX time (s)"=w838:dbl)  [unwired: 9 in]
        n338 = call "LV_UNIX.vi"("current time"=w845) -> ("date/time string"=w843:string, "UNIX time (s)"=w844:dbl)  [unwired: 9 in]
        n339 = Unbundle(w827) -> ("LSI-D out[0]"=w828:dbl, "LSI-D out[1]"=w829:dbl, "LSI-D out[2]"=w830:dbl, "LSI-D out[3]"=w831:dbl, "LSI-D out[4]"=w832:dbl, "LSI-D out[5]"=w833:dbl, "LSI-D out[6]"=w834:dbl, "LSI-D out[7]"=w835:dbl)  [unwired: 1 out]
        n340 = Unbundle(w856) -> ("LSI-U out[0]"=w855:dbl, "LSI-U out[1]"=w854:dbl, "LSI-U out[2]"=w853:dbl, "LSI-U out[3]"=w852:dbl, "LSI-U out[4]"=w851:dbl, "LSI-U out[5]"=w850:dbl, "LSI-U out[6]"=w849:dbl, "LSI-U out[7]"=w848:dbl)  [unwired: 1 out]
        n341 = Format Into String(format string="%d,%s,%10.4f,%10.4f,%5.6f,%5.6f,%5.6f,%5.6f,%5.6f,%5.6f,%5.6f,%5.6f\\n", initial string=w823, error in=w824, w840, w839, w838, w825, w828, w829, w830, w831, w832, w833, w834, w835) -> (error out=→"error out \n(record LSID)":errorcluster)  [unwired: 1 out]
        n342 = Format Into String(format string="%d,%s,%10.4f,%10.4f,%5.6f,%5.6f,%5.6f,%5.6f,%5.6f,%5.6f,%5.6f,%5.6f\\n", initial string=w861, error in=w860, w842, w843, w844, w859, w855, w854, w853, w852, w851, w850, w849, w848) -> (error out=→"error out \n(record LSIU)":errorcluster)  [unwired: 1 out]
      }
    }
    n343 = stacked-sequence {
      tunnel: w499 -> [w591 _]
      tunnel: w498 -> [_ w703]
      tunnel: [_ w701] -> w486
      tunnel: w497 -> [w569 _]
      tunnel: [w527 _] -> w491
      tunnel: w492 -> [w526 _]
      tunnel: [w568 _] -> w487
      tunnel: [_ w699] -> w485
      frame #0 {
        n344 = local read "NI DAQ AIN labels"() -> (→"NI-DAQ CH indic.":string[])
        n345 = local read "error out\n(DAQ config)"() -> (w587:errorcluster)
        n346 = local read "sample #"() -> (w564:i32)
        n347 = call <vilib>:"DAQmx Read (Analog 2D DBL NChan NSamp).vi"("task/channels in"=w591, "number of samples per channel"=w564, "timeout"=100.0, "error in"=w587) -> ("task out"=w568:refnum<k21>, "data"=w586:dbl[][], "error out"=→"error out \n(DAQ IN)":errorcluster)  [unwired: 9 in]
        n348 = Index Array(array=w586, index (row) #1=0 ("index (row)"), index (row) #2=1 ("index (row)"), index (row) #3=2 ("index (row)"), index (row) #4=3 ("index (row)"), index (row) #5=4 ("disabled index (col)"), index (row) #6=5 ("index (col)"), index (row) #7=6 ("disabled index (row)"), index (row) #8=7 ("disabled index (row)"), index (row) #9=8 ("disabled index (row)")) -> (element #1=w548:dbl[], element #2=w553:dbl[], element #3=w557:dbl[], element #4=w550:dbl[], element #5=w549:dbl[], element #6=w547:dbl[], element #7=w534:dbl[], element #8=w533:dbl[], element #9=w532:dbl[])  [unwired: 9 in]
        n349 = stacked-sequence {
          tunnel: [w626 _ _ _ _ _ _ _ _] -> w567
          tunnel: [_ w635 _ _ _ _ _ _ _] -> w565
          tunnel: w564 -> [_ w633 w643 w652 w661 w670 w679 w688 w697]
          tunnel: w564 -> [w624 _ _ _ _ _ _ _ _]
          tunnel: [_ _ w641 _ _ _ _ _ _] -> w563
          tunnel: w553 -> [_ w631 _ _ _ _ _ _ _]
          tunnel: [_ _ _ w650 _ _ _ _ _] -> w560
          tunnel: [_ _ _ _ w659 _ _ _ _] -> w559
          tunnel: [_ _ _ _ _ w668 _ _ _] -> w558
          tunnel: w557 -> [_ _ w640 _ _ _ _ _ _]
          tunnel: [_ _ _ _ _ _ w677 _ _] -> w556
          tunnel: w550 -> [_ _ _ w649 _ _ _ _ _]
          tunnel: w549 -> [_ _ _ _ w658 _ _ _ _]
          tunnel: w548 -> [w622 _ _ _ _ _ _ _ _]
          tunnel: w547 -> [_ _ _ _ _ w667 _ _ _]
          tunnel: w534 -> [_ _ _ _ _ _ w676 _ _]
          tunnel: w533 -> [_ _ _ _ _ _ _ w682 _]
          tunnel: w532 -> [_ _ _ _ _ _ _ _ w691]
          tunnel: [_ _ _ _ _ _ _ w681 _] -> w531
          tunnel: [_ _ _ _ _ _ _ _ w690] -> w530
          frame #0 {
            # "P (4K)"
            n350 = Add Array Elements(numeric array=w622) -> (sum=w625:dbl)
            n351 = Divide(x=w625, y=w624) -> (x/y=w623:dbl)
            n352 = call "scaling_calculator.vi"("x1"=1.0, "y1"=0.0 ("x1"), "x"=w623, "x2"=3.0 ("x1"), "y2"=100000.0 ("x1")) -> ("y"=w626:dbl)  [unwired: 2 in]
          }
          frame #1 {
            # "LM"
            n353 = Add Array Elements(numeric array=w631) -> (sum=w634:dbl)
            n354 = Divide(x=w634, y=w633) -> (x/y=w632:dbl)
            n355 = call "scaling_calculator.vi"("x1"=0.0, "y1"=0.0 ("x1"), "x"=w632, "x2"=0.1 ("x1"), "y2"=100.0 ("x1")) -> ("y"=w635:dbl)  [unwired: 2 in]
          }
          frame #2 {
            # "Delta P He 4"
            n356 = Add Array Elements(numeric array=w640) -> (sum=w644:dbl)
            n357 = Divide(x=w644, y=w643) -> (x/y=w642:dbl)
            n358 = call "scaling_calculator.vi"("x1"=1.0, "y1"=0.0 ("x1"), "x"=w642, "x2"=5.0 ("x1"), "y2"=1000.0 ("x1")) -> ("y"=w641:dbl)  [unwired: 2 in]
          }
          frame #3 {
            # "Delta P He 3"
            n359 = Add Array Elements(numeric array=w649) -> (sum=w653:dbl)
            n360 = Divide(x=w653, y=w652) -> (x/y=w651:dbl)
            n361 = call "scaling_calculator.vi"("x1"=1.0, "y1"=0.0 ("x1"), "x"=w651, "x2"=5.0 ("x1"), "y2"=1000.0 ("x1")) -> ("y"=w650:dbl)  [unwired: 2 in]
          }
          frame #4 {
            # "FM He4"
            n362 = Add Array Elements(numeric array=w658) -> (sum=w662:dbl)
            n363 = Divide(x=w662, y=w661) -> (x/y=w660:dbl)
            n364 = call "scaling_calculator.vi"("x1"=0.0, "y1"=0.0 ("x1"), "x"=w660, "x2"=5.0 ("x1"), "y2"=500.0 ("x1")) -> ("y"=w659:dbl)  [unwired: 2 in]
          }
          frame #5 {
            # "FM He3"
            n365 = Add Array Elements(numeric array=w667) -> (sum=w671:dbl)
            n366 = Divide(x=w671, y=w670) -> (x/y=w669:dbl)
            n367 = call "scaling_calculator.vi"("x1"=0.0, "y1"=0.0 ("x1"), "x"=w669, "x2"=5.0 ("x1"), "y2"=200.0 ("x1")) -> ("y"=w668:dbl)  [unwired: 2 in]
          }
          frame #6 {
            # "BARATRON"
            n368 = Add Array Elements(numeric array=w676) -> (sum=w680:dbl)
            n369 = Divide(x=w680, y=w679) -> (x/y=w678:dbl)
            n370 = call "scaling_calculator_baratron.vi"("x"=w678) -> ("y (Pa)"=w677:dbl)  [unwired: 5 in, 1 out]
          }
          frame #7 {
            # "AI16 P 4He IN"
            n371 = Add Array Elements(numeric array=w682) -> (sum=w689:dbl)
            n372 = Divide(x=w689, y=w688) -> (x/y=w683:dbl)
            n373 = call "scaling_calculator.vi"("x1"=1.0, "y1"=0.0 ("x1"), "x"=w683, "x2"=5.0 ("x1"), "y2"=200000.0 ("x1")) -> ("y"=w681:dbl)  [unwired: 2 in]
          }
          frame #8 {
            # "AI17 P 3He OUT"
            n374 = Add Array Elements(numeric array=w691) -> (sum=w698:dbl)
            n375 = Divide(x=w698, y=w697) -> (x/y=w692:dbl)
            n376 = call "scaling_calculator.vi"("x1"=1.0, "y1"=0.0 ("x1"), "x"=w692, "x2"=5.0 ("x1"), "y2"=200000.0 ("x1")) -> ("y"=w690:dbl)  [unwired: 2 in]
          }
        }
        n377 = Build Array(w567, w565, w563, w560, w559, w558, w556, w531, w530) -> (w544:dbl[])
        "NI DAQ OUT" <- w544
        n378 = local read "current time"() -> (w524:timestamp)
        n379 = local read "error out\n(file creation)"() -> (w583:errorcluster)
        n380 = Build Array (concatenate)(w569, w544) -> (w527:dbl[][])
        n381 = Array To Cluster(array=w544) -> (cluster=w546:T8)
        n382 = local read "ref DAQ"() -> (w582:refnum<file>)
        n383 = local read "Cycle #"() -> (w521:i32)
        n384 = To Double Precision Float(number=w524) -> (double precision float=w584:dbl)
        n385 = call "LV_UNIX.vi"("current time"=w524) -> ("date/time string"=w522:string, "UNIX time (s)"=w523:dbl)  [unwired: 9 in]
        n386 = Unbundle(w546) -> ("[0]"=w545:dbl, "[1]"=w543:dbl, "[2]"=w542:dbl, "[3]"=w541:dbl, "[4]"=w540:dbl, "[5]"=w539:dbl, "[6]"=w538:dbl, "[7]"=w529:dbl, "[8]"=w528:dbl)
        n387 = Index Array(array=w527, index (col) #1=0 ("disabled index (col)"), index (col) #2=1 ("disabled index (col)"), index (col) #3=2 ("disabled index (col)"), index (col) #4=3 ("disabled index (col)"), index (col) #5=4 ("index (col)"), index (col) #6=5 ("index (col)"), index (col) #7=6 ("index (col)"), index (col) #8=7 ("index (col)"), index (col) #9=8 ("index (col)")) -> (element #1=w580:dbl[], element #2=w578:dbl[], element #3=w576:dbl[], element #4=w574:dbl[], element #5=w571:dbl[], element #6=w570:dbl[], element #7=w554:dbl[], element #8=w516:dbl[], element #9=w515:dbl[])  [unwired: 9 in]
        n388 = Format Into String(format string="%d,%s,%10.4f,%10.4f,%5.6f,%5.6f,%5.6f,%5.6f,%5.6f,%5.6f,%5.6f,%5.6f,%5.6f\\n", initial string=w582, error in=w583, w521, w522, w523, w584, w545, w543, w542, w541, w540, w539, w538, w529, w528) -> (error out=→"error out \n(record DAQ)":errorcluster)  [unwired: 1 out]
        n389 = Bundle(w526, w580) -> (w520:cluster{dbl[], dbl[]})  [unwired: 1 in]
        n390 = Bundle(w526, w578) -> (w519:cluster{dbl[], dbl[]})  [unwired: 1 in]
        n391 = Bundle(w526, w576) -> (w514:cluster{dbl[], dbl[]})  [unwired: 1 in]
        n392 = Bundle(w526, w574) -> (w513:cluster{dbl[], dbl[]})  [unwired: 1 in]
        n393 = Bundle(w526, w571) -> (w512:cluster{dbl[], dbl[]})  [unwired: 1 in]
        n394 = Bundle(w526, w570) -> (w511:cluster{dbl[], dbl[]})  [unwired: 1 in]
        n395 = Bundle(w526, w516) -> (w510:cluster{dbl[], dbl[]})  [unwired: 1 in]
        n396 = Bundle(w526, w554) -> (w509:cluster{dbl[], dbl[]})  [unwired: 1 in]
        n397 = Bundle(w526, w515) -> (w507:cluster{dbl[], dbl[]})  [unwired: 1 in]
        n398 = Build Array(w520, w519, w514, w513, w512, w511, w510, w509, w507) -> (w506:cluster{dbl[], dbl[]}[])
        n399 = stacked-sequence {
          tunnel: w506 -> [w594 w600 w605 w610 w615 w620]
          frame #0 {
            n400 = control-ref of="Graph S. 1"() -> (w595:refnum<vi>)
            n401 = property class="XYGraph (strict)"(reference=w595, error in=errorcluster {"status"=FALSE, "code"=0, "source"=""} ("error in (no error)"), "Value"=w594) -> (error out=w592:errorcluster)  [unwired: 1 out]
            n402 = control-ref of="error plot content"() -> (w593:refnum<vi>)
            n403 = property class="Clust (strict)"(reference=w593, "Value"=w592) -> ()  [unwired: 1 in, 2 out]
          }
          frame #1 {
            n404 = control-ref of="Graph S. 2"() -> (w597:refnum<vi>)
            n405 = property class="XYGraph (strict)"(reference=w597, error in=errorcluster {"status"=FALSE, "code"=0, "source"=""} ("error in (no error)"), "Value"=w600) -> (error out=w598:errorcluster)  [unwired: 1 out]
            n406 = control-ref of="error plot content"() -> (w599:refnum<vi>)
            n407 = property class="Clust (strict)"(reference=w599, "Value"=w598) -> ()  [unwired: 1 in, 2 out]
          }
          frame #2 {
            n408 = control-ref of="Graph S. 3"() -> (w602:refnum<vi>)
            n409 = property class="XYGraph (strict)"(reference=w602, error in=errorcluster {"status"=FALSE, "code"=0, "source"=""} ("error in (no error)"), "Value"=w605) -> (error out=w603:errorcluster)  [unwired: 1 out]
            n410 = control-ref of="error plot content"() -> (w604:refnum<vi>)
            n411 = property class="Clust (strict)"(reference=w604, "Value"=w603) -> ()  [unwired: 1 in, 2 out]
          }
          frame #3 {
            n412 = control-ref of="Graph S. 4"() -> (w607:refnum<vi>)
            n413 = property class="XYGraph (strict)"(reference=w607, error in=errorcluster {"status"=FALSE, "code"=0, "source"=""} ("error in (no error)"), "Value"=w610) -> (error out=w608:errorcluster)  [unwired: 1 out]
            n414 = control-ref of="error plot content"() -> (w609:refnum<vi>)
            n415 = property class="Clust (strict)"(reference=w609, "Value"=w608) -> ()  [unwired: 1 in, 2 out]
          }
          frame #4 {
            n416 = control-ref of="Graph S. 5"() -> (w612:refnum<vi>)
            n417 = property class="XYGraph (strict)"(reference=w612, error in=errorcluster {"status"=FALSE, "code"=0, "source"=""} ("error in (no error)"), "Value"=w615) -> (error out=w613:errorcluster)  [unwired: 1 out]
            n418 = control-ref of="error plot content"() -> (w614:refnum<vi>)
            n419 = property class="Clust (strict)"(reference=w614, "Value"=w613) -> ()  [unwired: 1 in, 2 out]
          }
          frame #5 {
            n420 = control-ref of="Graph S. 6"() -> (w617:refnum<vi>)
            n421 = property class="XYGraph (strict)"(reference=w617, error in=errorcluster {"status"=FALSE, "code"=0, "source"=""} ("error in (no error)"), "Value"=w620) -> (error out=w618:errorcluster)  [unwired: 1 out]
            n422 = control-ref of="error plot content"() -> (w619:refnum<vi>)
            n423 = property class="Clust (strict)"(reference=w619, "Value"=w618) -> ()  [unwired: 1 in, 2 out]
          }
        }
      }
      frame #1 {
        n424 = local read "error out \n(DAQ IN)"() -> (w700:errorcluster)
        n425 = local read "DAQ OUT ON?"() -> (w702:bool)
        n426 = case shown="True" w702 {
          tunnel: w703 -> [w705 w710]
          tunnel: [w705 w709] -> w701
          tunnel: w700 -> [w704 w707]
          tunnel: [w704 w706] -> w699
          frame False {
          }
          frame True {
            n427 = call <vilib>:"DAQmx Write (Analog 1D DBL 1Chan NSamp).vi"("task/channels in"=w710, "data"="DAQ OUT SET Volt", "timeout"=100.0, "error in"=w707) -> ("task out"=w709:refnum<k21>, "number of samples written per channel"=→"DAQ OUT \nsample #":u32, "error out"=w706:errorcluster)  [unwired: 9 in]
          }
        }
        "error out\n(DAQ OUT)" <- w699
      }
    }
    "Cycle #" <- w500
  }
  n428 = call <vilib>:"DAQmx Stop Task.vi"("task/channels in"=w12, "error in"=w10) -> ("task out"=w14:refnum<k21>, "error out"=w13:errorcluster)  [unwired: 12 in]
  n429 = call <vilib>:"DAQmx Clear Task.vi"("task in"=w14, "error in"=w13) -> ("error out"=w16:errorcluster)  [unwired: 13 in]
  n430 = call <vilib>:"DAQmx Stop Task.vi"("task/channels in"=w11, "error in"=w16) -> ("task out"=w18:refnum<k21>, "error out"=w15:errorcluster)  [unwired: 12 in]
  n431 = call <vilib>:"DAQmx Clear Task.vi"("task in"=w18, "error in"=w15) -> ("error out"=→"error out DAQ close":errorcluster)  [unwired: 13 in]
